vi "ReCalc.vi"(3 "Berechnen":bool, 4 "Datenspeicher":T3={"Fahrzeugdaten"="§$", "Auto-Pfad"="21.01.2021 18:54|N:\\Vespa-Prüfstand\\Läufe\\Test", "Rolle [Inkr/U]"=100, "Rollenumfang [m]"=0.942, "Rollenträgheit [kgm²]"=0.164, "Zündung [Imp/U]"=1.0, "Getriebe [1:]"=4.0, "Reifenumfang [m] "=1.222, "element"=3.988, "Gl. Mittelwert"=35, "Differenzenquotient"=12, "AFR, EGT"=1, "dT [s]"=0.02, "Strecke [m]"=150.92789069243696, "Lufttemperatur [°C]"=23.2, "Mv: n1 [1/min]"=1.0, "Luftdruck [mbar]"=100.34, "nRolle"=array[576 elements], "nWelle"=array[576 elements], "AFR"=[14.9, 14.9, 14.9, 14.9, 14.9, 14.9, 14.9, 14.9, 14.9, 14.9, 15.4, 15.4, 15.4, 15.4, 15.4, 14.8, 14.8, 14.8, 14.8, 14.8, 15.3, 15.3, 15.3, 15.3, 15.3, 15.2, 15.2, 15.2, 15.2, 15.2, 14.8, 14.8, 14.8, 14.8, 14.8, 15.0, 15.0, 15.0, 15.0, 15.0, 15.0, 15.0, 15.0, 15.0, 15.0, 15.0, 15.0, 15.0, 15.0, 15.0, 15.0, 15.0, 15.0, 15.0, 15.0, 15.4, 15.4, 15.4, 15.4, 15.4, 15.4, 15.4, 15.4, 15.4, 15.4, 14.9, 14.9, 14.9, 14.9, 14.9, 15.3, 15.3, 15.3, 15.3, 15.3, 15.0, 15.0, 15.0, 15.0, 15.0, 14.8, 14.8, 14.8, 14.8, 14.8, 15.2, 15.2, 15.2, 15.2, 15.2, 15.4, 15.4, 15.4, 15.4, 15.4, 15.1, 15.1, 15.1, 15.1, 15.1, 15.1, 15.1, 15.1, 15.1, 15.1, 15.1, 15.1, 15.1, 15.1, 15.1, 15.0, 15.0, 15.0, 15.0, 15.0, 15.0, 15.0, 15.0, 15.0, 15.0, 15.2, 15.2, 15.2, 15.2, 15.2, 15.1, 15.1, 15.1, 15.1, 15.1, 15.4, 15.4, 15.4, 15.4, 15.4, 15.1, 15.1, 15.1, 15.1, 15.1, 15.2, 15.2, 15.2, 15.2, 15.2, 14.8, 14.8, 14.8, 14.8, 14.8, 15.4, 15.4, 15.4, 15.4, 15.4, 15.0, 15.0, 15.0, 15.0, 15.0, 15.1, 15.1, 15.1, 15.1, 15.1, 15.0, 15.0, 15.0, 15.0, 15.0, 15.1, 15.1, 15.1, 15.1, 15.1, 14.9, 14.9, 14.9, 14.9, 14.9, 15.0, 15.0, 15.0, 15.0, 15.0, 15.2, 15.2, 15.2, 15.2, 15.2, 15.3, 15.3, 15.3, 15.3, 15.3, 15.1, 15.1, 15.1, 15.1, 15.1, 15.1, 15.1, 15.1, 15.1, 15.1, 14.9, 14.9, 14.9, 14.9, 14.9, 15.0, 15.0, 15.0, 15.0, 15.0, 15.3, 15.3, 15.3, 15.3, 15.3, 15.3, 15.3, 15.3, 15.3, 15.3, 15.1, 15.1, 15.1, 15.1, 15.1, 15.4, 15.4, 15.4, 15.4, 15.4, 15.0, 15.0, 15.0, 15.0, 15.0, 14.9, 14.9, 14.9, 14.9, 14.9, 15.0, 15.0, 15.0, 15.0, 15.0, 15.3, 15.3, 15.3, 15.3, 15.3, 15.0, 15.0, 15.0, 15.0, 15.0, 14.9, 14.9, 14.9, 14.9, 14.9, 14.9, 14.9, 14.9, 14.9, 14.9, 15.4, 15.4, 15.4, 15.4, 15.4, 15.1, 15.1, 15.1, 15.1, 15.1, 15.2, 15.2, 15.2, 15.2, 15.2, 15.2, 15.2, 15.2, 15.2, 15.2, 15.1, 15.1, 15.1, 15.1, 15.1, 15.4, 15.4, 15.4, 15.4, 15.4, 15.3, 15.3, 15.3, 15.3, 15.3, 14.9, 14.9, 14.9, 14.9, 14.9, 15.4, 15.4, 15.4, 15.4, 15.4, 15.1, 15.1, 15.1, 15.1, 15.1, 15.2, 15.2, 15.2, 15.2, 15.2, 15.2, 15.2, 15.2, 15.2, 15.2, 15.3, 15.3, 15.3, 15.3, 15.3, 14.9, 14.9, 14.9, 14.9, 14.9, 15.3, 15.3, 15.3, 15.3, 15.3, 14.9, 14.9, 14.9, 14.9, 14.9, 14.9, 14.9, 14.9, 14.9, 14.9, 15.1, 15.1, 15.1, 15.1, 15.1, 15.1, 15.1, 15.1, 15.1, 15.1, 15.3, 15.3, 15.3, 15.3, 15.3, 15.3, 15.3, 15.3, 15.3, 15.3, 15.0, 15.0, 15.0, 15.0, 15.0, 15.1, 15.1, 15.1, 15.1, 15.1, 15.2, 15.2, 15.2, 15.2, 15.2, 15.1, 15.1, 15.1, 15.1, 15.1, 15.4, 15.4, 15.4, 15.4, 15.4, 15.0, 15.0, 15.0, 15.0, 15.0, 15.4, 15.4, 15.4, 15.4, 15.4, 15.4, 15.4, 15.4, 15.4, 15.4, 15.1, 15.1, 15.1, 15.1, 15.1, 15.1, 15.1, 15.1, 15.1, 15.1, 15.0, 15.0, 15.0, 15.0, 15.0, 15.1, 15.1, 15.1, 15.1, 15.1, 15.1, 15.1, 15.1, 15.1, 15.1, 15.1, 15.1, 15.1, 15.1, 15.1, 15.2, 15.2, 15.2, 15.2, 15.2, 14.9, 14.9, 14.9, 14.9, 14.9, 15.2, 15.2, 15.2, 15.2, 15.2, 15.3, 15.3, 15.3, 15.3, 15.3, 15.3, 15.3, 15.3, 15.3, 15.3, 15.3, 15.3, 15.3, 15.3, 15.3, 14.9, 14.9, 14.9, 14.9, 14.9, 14.9, 14.9, 14.9, 14.9, 14.9, 15.1, 15.1, 15.1, 15.1, 15.1, 15.0, 15.0, 15.0, 15.0, 15.0, 15.4, 15.4, 15.4, 15.4, 15.4, 15.2, 15.2, 15.2, 15.2, 15.2, 15.1, 15.1, 15.1, 15.1, 15.1, 15.0, 15.0, 15.0, 15.0, 15.0, 15.1, 15.1, 15.1, 15.1, 15.1, 15.4, 15.4, 15.4, 15.4, 15.4, 15.0, 15.0, 15.0, 15.0, 15.0, 15.2, 15.2, 15.2, 15.2, 15.2, 14.9, 14.9, 14.9, 14.9, 14.9, 15.3, 15.3, 15.3, 15.3, 15.3, 14.9, 14.9, 14.9, 14.9, 14.9, 14.9, 14.9, 14.9, 14.9, 14.9, 15.0, 15.0, 15.0, 15.0, 15.0, 15.2, 15.2, 15.2, 15.2, 15.2, 15.0, 15.0, 15.0, 15.0, 15.0, 15.2, 15.2, 15.2, 15.2, 15.2, 15.2], "EGT"=array[576 elements], "Übersetzung ermitteln aus"=0, "[s]"=5.0, "Mv: M0 [Nm]"=0.0, "Mv: M1 [Nm]"=0.0, "n vom Gas [1/min]"=5000.0, "dT ungefiltert [s]"=array[576 elements], [], "Boolesch"=TRUE, "Serielle Schnittstelle"="", "nKuWe/nRolle 2"=3.988, "v vom Gas [km/h]"=40.0}) -> ()   [LabVIEW 2014]
uses:
  <vilib>/Utility/miscctls.llb/LVPointTypeDef.ctl
  <vilib>/Analysis/3filter.llb/IIR Filter (DBL).vi
  <vilib>/Analysis/NI_AALBase.lvlib
panel:
  in  "Resetskalierung Leistung":bool
  out "Y-Koord. Leistungsgraph-Reset-Button oben (567)":i32=567
  out "Y-Koord. Leistungsgraph-Reset-Button unten (782)":i32=782
  in  "Autoskalierung Leistung":bool
  in  "Resetskalierung AFR":bool
  in  "Autoskalierung AFR":bool
  out "EGT [°C]":dbl
  out "CursorAFR - Beschriftung":string="AFR"
  out "AFR":dbl format="%.1f"
  out "Fahrzeugdaten":string
  out "Ergebnis":string
  in  "Lambda":bool caption="Messung Klimadaten"
  in  "AFR, EGT":bool caption="Messung Klimadaten"
  out "Höhe Leistungs-Graph (646)":u32=646
  in  "title diagram":string
  out "Strecken":T1 {"Strecke7" scale=0.0..200.0; "Strecke6" scale=0.0..200.0; "Strecke5" scale=0.0..200.0; "Strecke4" scale=0.0..200.0; "Strecke3" scale=0.0..200.0; "Strecke2" scale=0.0..200.0; "Strecke1" max=600.0 scale=0.0..200.0}
  out "Dateiname":string
  out "Datum+Zeit":string="21.01.2021 18:54"
  out "Elementindex":dbl
  in  "Mv: M1 [Nm]":dbl min=0.0
  in  "Mv: M0 [Nm]":dbl min=0.0
  in  "Mv: n1 [1/min]":u16=1 min=1
  out "Überlagerung":bool
  out "CursorY2 - Beschriftung":string="M [Nm]"
  out "CursorX - Beschriftung":string="n [1/min]"
  out "M [Nm]":dbl format="%#.1f"
  out "P [PS]":dbl format="%#.1f"
  out "n [1/min]":dbl caption="n {1/min]" format="%#.0f"
  in  "v min [km/h]":dbl=40.0
  in  "Legende einblenden":bool=TRUE
  in  "Überlagern":bool
  out "Übersetzung ermitteln aus":T2(ring)
  in  "Speichern":bool
  out "circum. tire [m]":dbl=1.222
  out "gear ratio [1:]":dbl=4.0
  out "ignition [Imp/U]":dbl=1.0
  out "incre./rev.  [Inkr/U]":u16=100
  out "air pressure [mbar]":dbl=100.34
  out "air temp. [°C]":dbl=23.2
  in  "Stopp":bool
  in  "inertia dyno [kgm²]":dbl=0.164
  in  "mov. Average":u8=35
  in  "diff.quotient":u8=12
  in  "n min [1/min]":dbl=5000.0
  out "circum. dyno [m]":dbl=0.942 format="%.3f"
  out "gear ratio from:":dbl=3.988 format="%.2f"
  in  "Drucken":bool
  out "Pmax":string
  in  "Öffnen":bool
  out "korr":dbl=3.988
  out "XY-Graph":cluster{dbl[], dbl[]}[](graph)
  out "AFR,EGT-Graph":cluster{dbl[], dbl[]}[](graph)
  # "AFR / l &  EGT"
  # "Elementindex des Button \"Überlagern\" variierte zw. 24 und 25 nach Hinzufügen/Löschen anderer Objekte.\nKann hier abgefragt werden und im Case dann entsprechend eingetragen werden."
  # "AFR <> l"
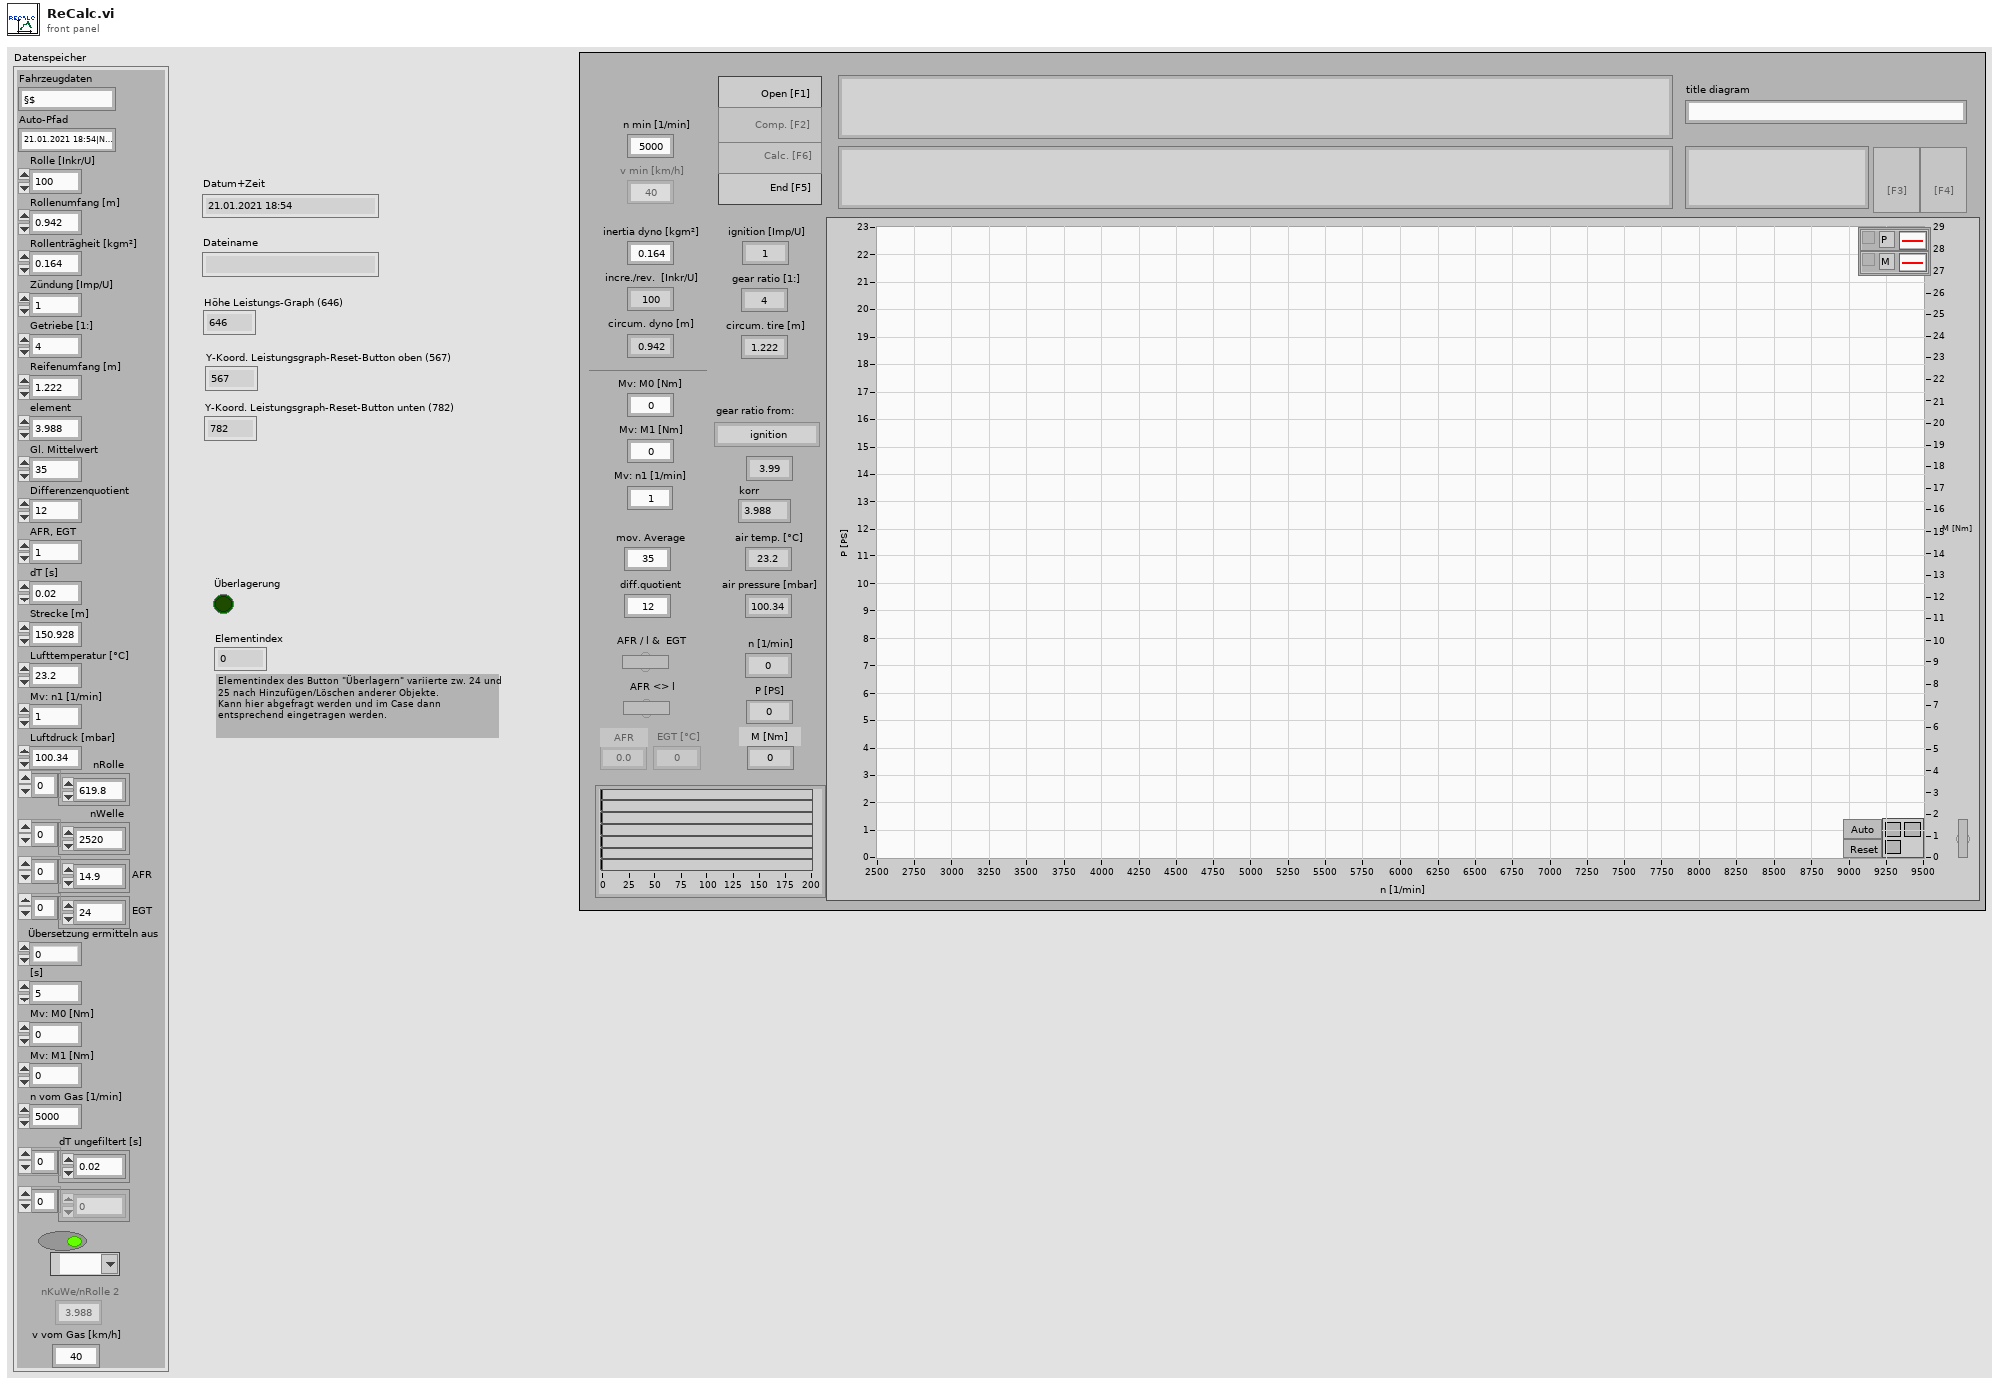
[diagram p1: front panel]
types:
  T1 = cluster{"Strecke1":dbl, "Strecke2":dbl, "Strecke3":dbl, "Strecke4":dbl, "Strecke5":dbl, "Strecke6":dbl, "Strecke7":dbl}
  T2 = enum8{"ignition ", "gear ratio & tire", "nCrank / nDyno", "vario [km/h]"}
  T3 = cluster{"Fahrzeugdaten":string, "Auto-Pfad":string, "Rolle [Inkr/U]":u16, "Rollenumfang [m]":dbl, "Rollenträgheit [kgm²]":dbl, "Zündung [Imp/U]":dbl, "Getriebe [1:]":dbl, "Reifenumfang [m] ":dbl, "element":dbl, "Gl. Mittelwert":u8, "Differenzenquotient":u8, "AFR, EGT":u8, "dT [s]":dbl, "Strecke [m]":dbl, "Lufttemperatur [°C]":dbl, "Mv: n1 [1/min]":dbl, "Luftdruck [mbar]":dbl, "nRolle":dbl[], "nWelle":dbl[], "AFR":dbl[], "EGT":dbl[], "Übersetzung ermitteln aus":u8, "[s]":dbl, "Mv: M0 [Nm]":dbl, "Mv: M1 [Nm]":dbl, "n vom Gas [1/min]":dbl, "dT ungefiltert [s]":dbl[], i32[], "Boolesch":bool, "Serielle Schnittstelle":refnum<visa-resource-name>, "nKuWe/nRolle 2":dbl, "v vom Gas [km/h]":dbl}
  T4 = typedef "LVPointTypeDef.ctl" = cluster{"Horizontal":i16, "Vertical":i16}
  T5 = enum8{"Enabled", "Disabled", "Disabled and Grayed Out"}
  T6 = cluster{"Fahrzeugdaten":string, "Auto-Pfad":string, "Rolle [Inkr/U]":u16, "Rollenumfang [m]":dbl, "Rollenträgheit [kgm²]":dbl, "Zündung [Imp/U]":dbl, "Getriebe [1:]":dbl, "Reifenumfang [m] ":dbl, "element":dbl, "Gl. Mittelwert":u8, "Differenzenquotient":u8, u8, "dT [s]":dbl, "Strecke [m]":dbl, "Lufttemperatur [°C]":dbl, "Mv: n1 [1/min]":dbl, "Luftdruck [mbar]":dbl, "nRolle":dbl[], "nWelle":dbl[], "AFR":dbl[], "EGT":dbl[], "Übersetzung ermitteln aus":u8, "[s]":dbl, "Mv: M0 [Nm]":dbl, "Mv: M1 [Nm]":dbl, "n vom Gas [1/min]":dbl, "dT-Array [s]":dbl[], i32[], "Boolesch":bool, "Serielle Schnittstelle":refnum<visa-resource-name>, "nKuWe/nRolle":dbl, "v vom Gas [km/h]":dbl}
  T7 = enum16{"Zündsignal", "Getriebe & Reifen", "nKuWe / nRolle", "Vario (km/h)"}
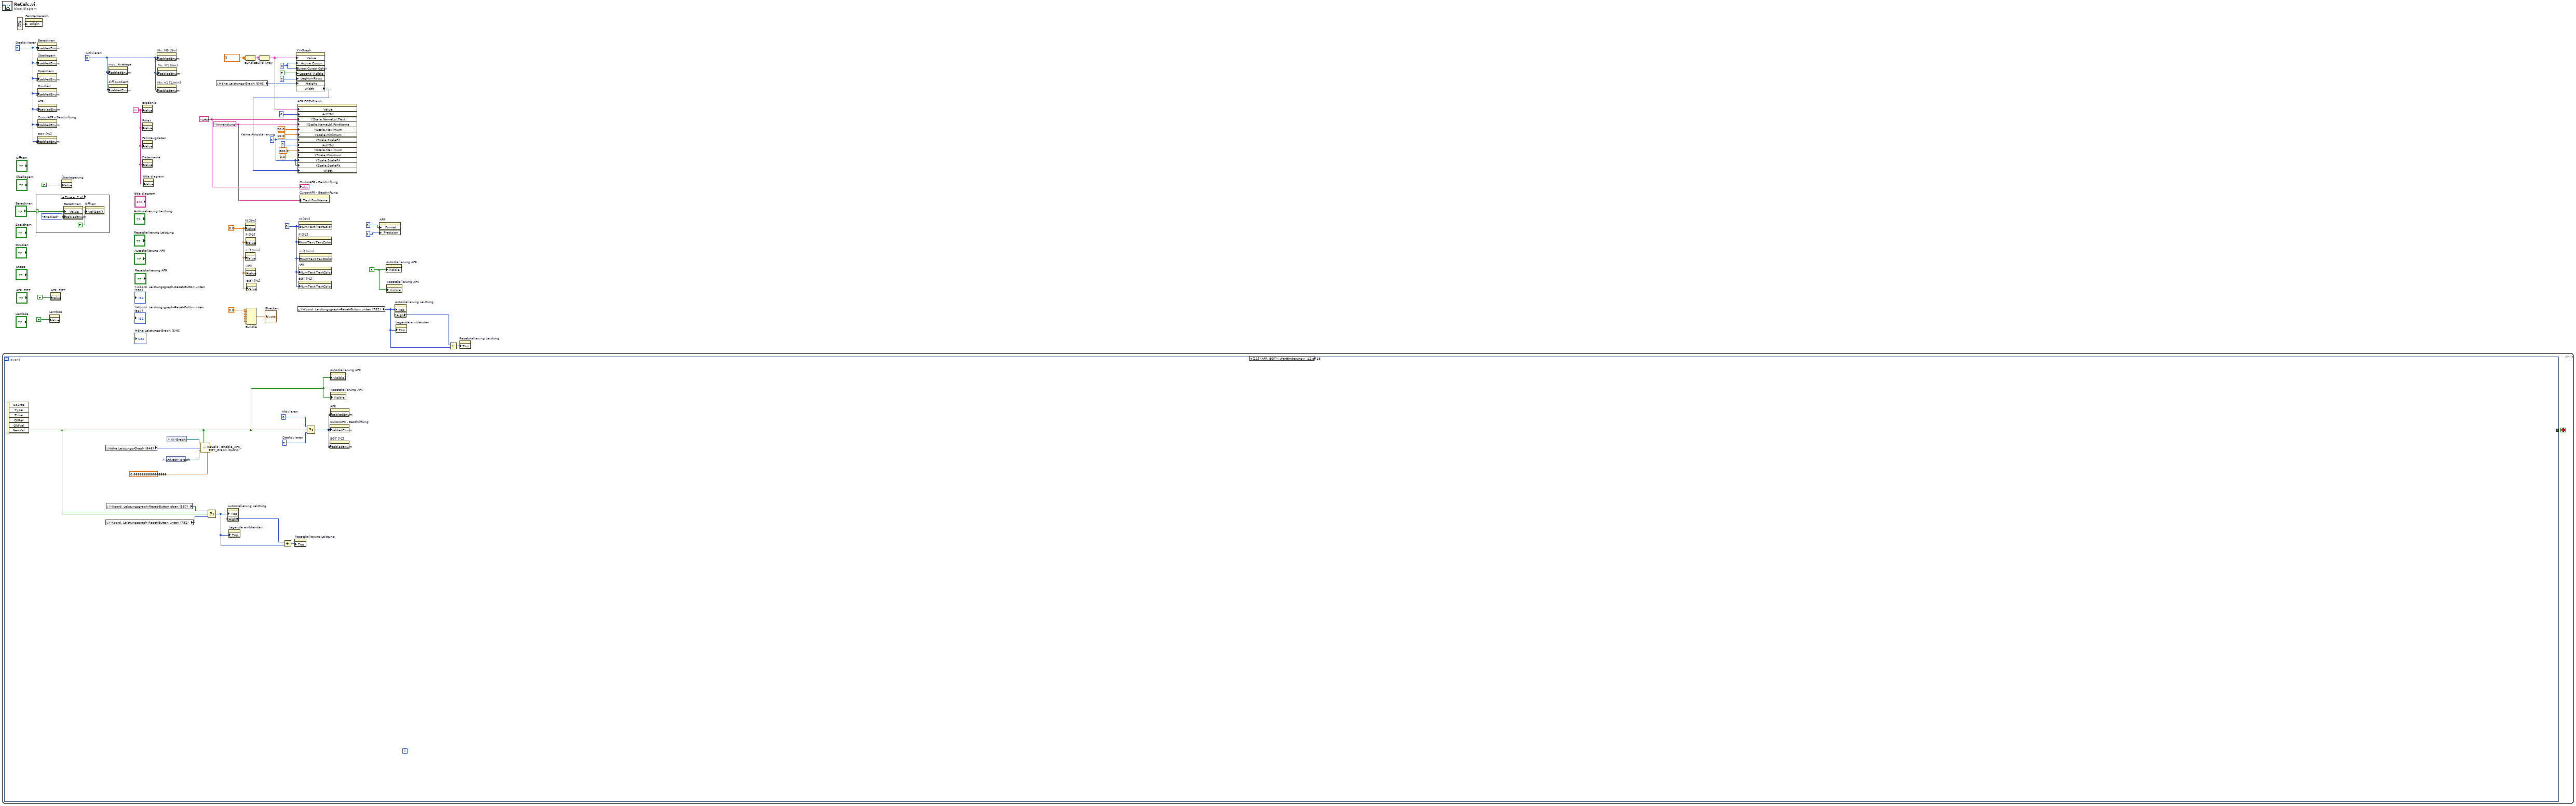
[diagram p0: block diagram]
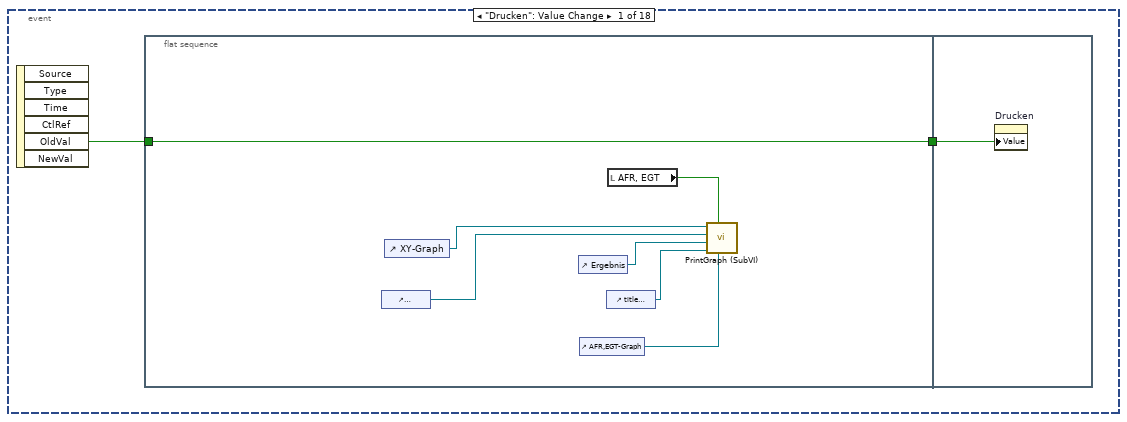
[diagram p3: hidden frame]
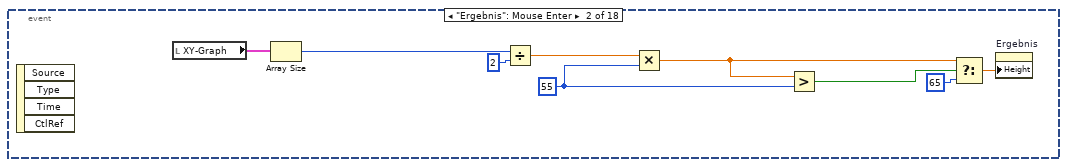
[diagram p4: hidden frame]
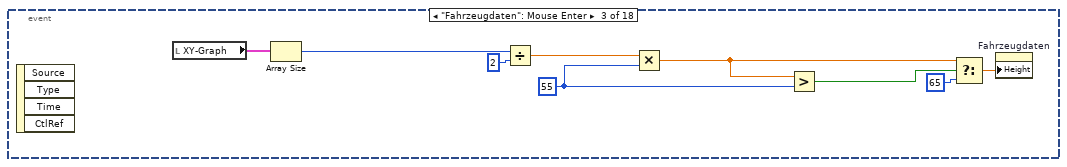
[diagram p5: hidden frame]
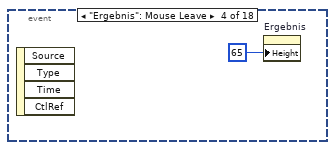
[diagram p6: hidden frame]
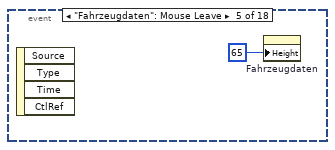
[diagram p7: hidden frame]
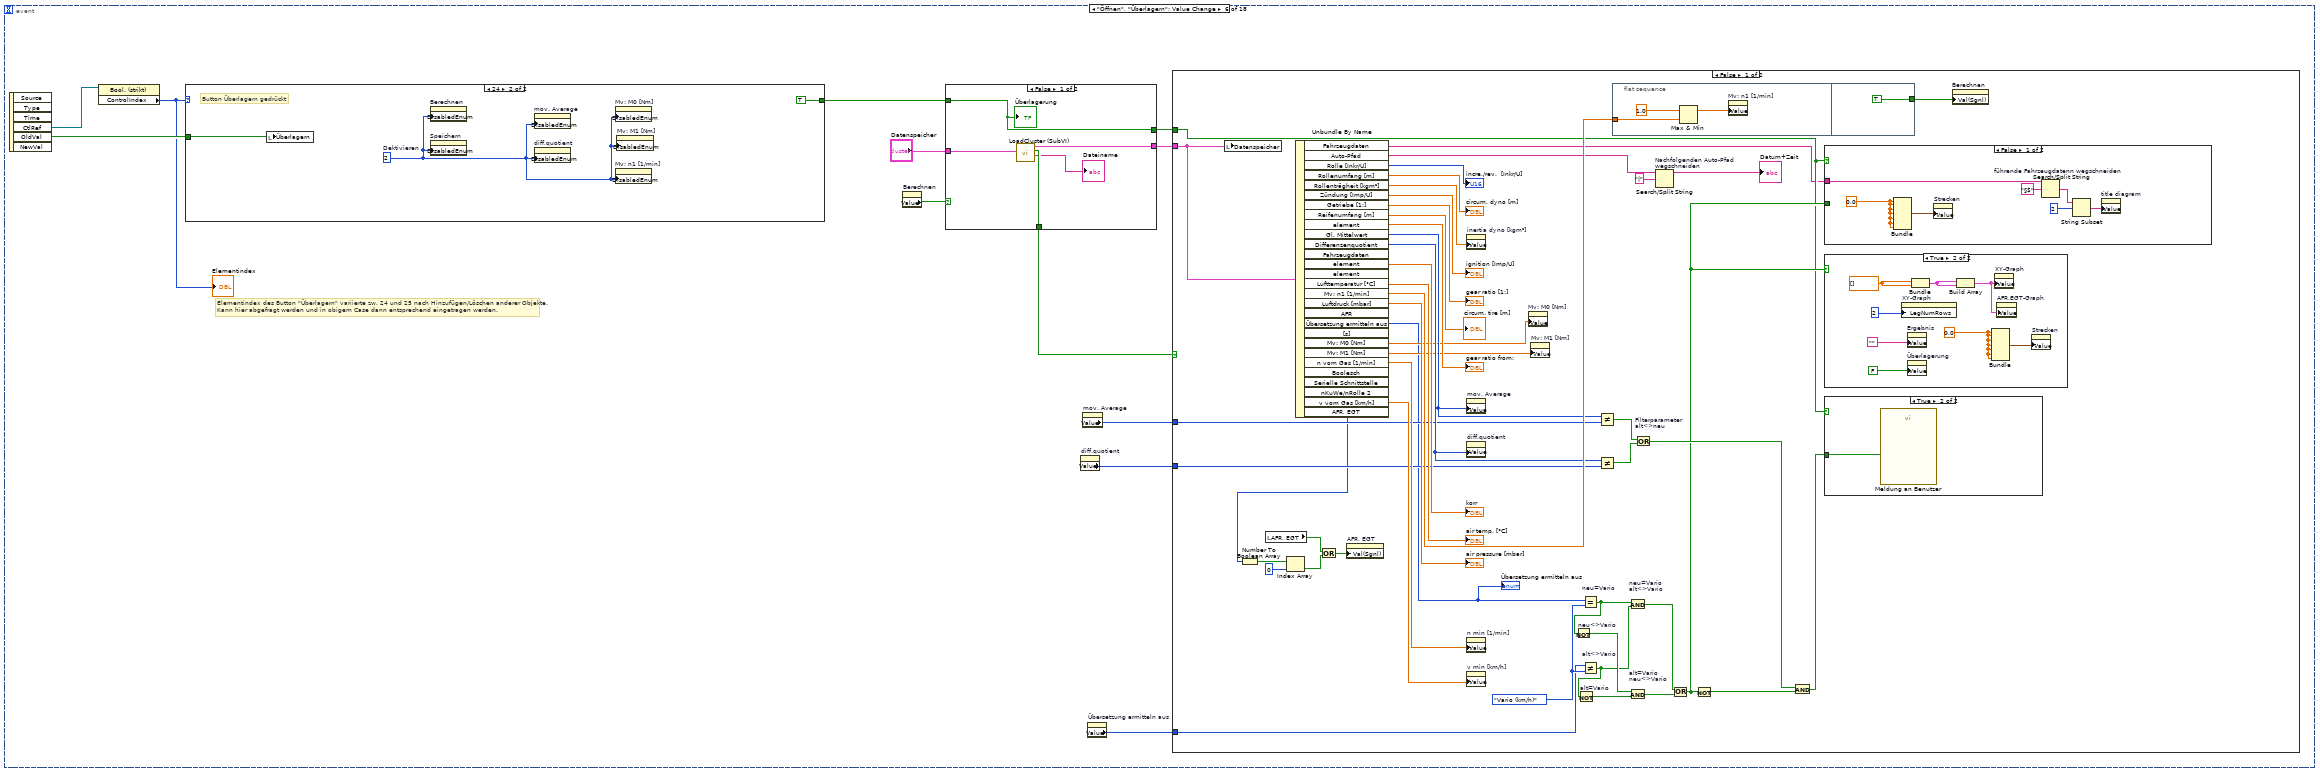
[diagram p8: hidden frame]
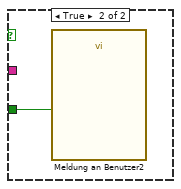
[diagram p10: hidden frame]
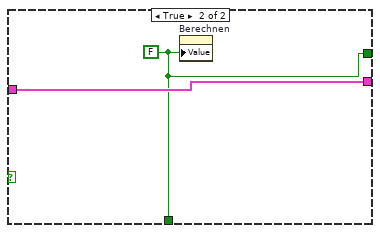
[diagram p13: hidden frame]
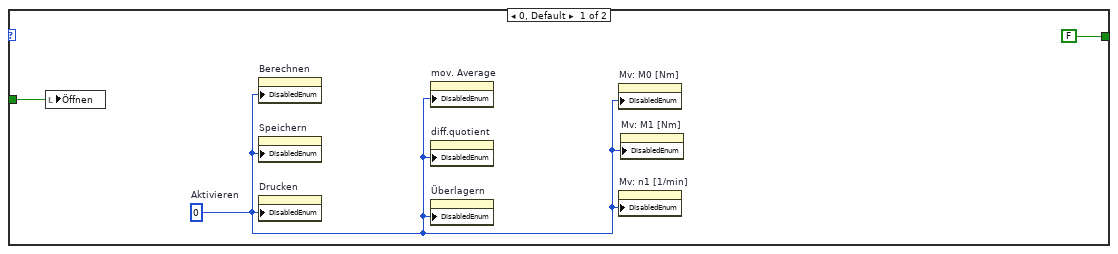
[diagram p14: hidden frame]
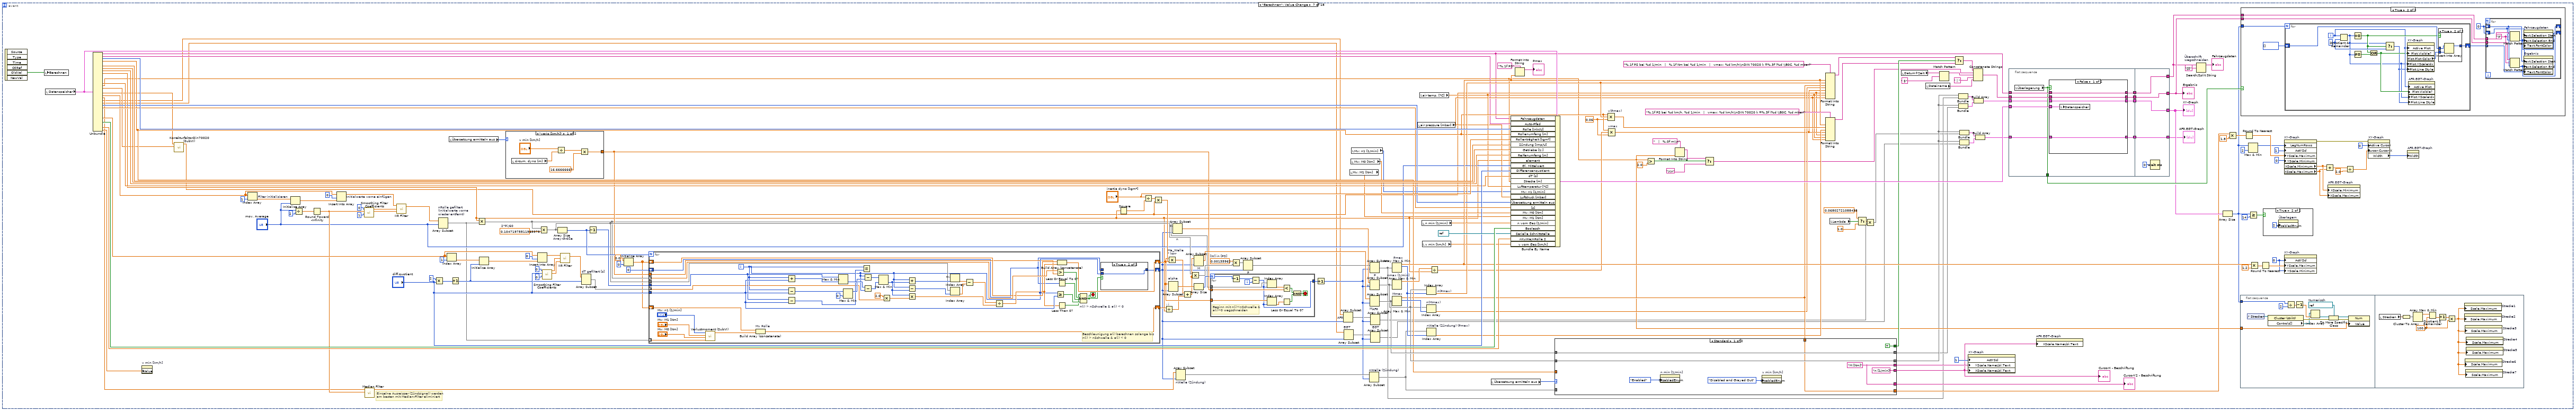
[diagram p15: hidden frame]
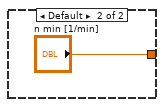
[diagram p16: hidden frame]
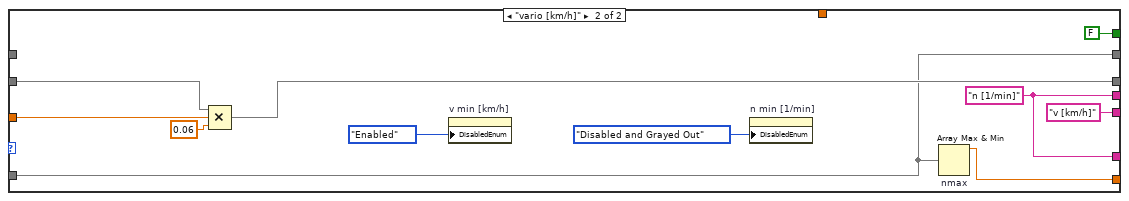
[diagram p17: hidden frame]
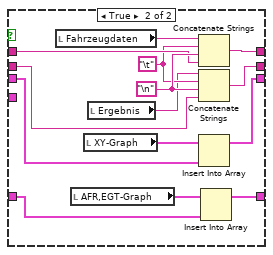
[diagram p19: hidden frame]
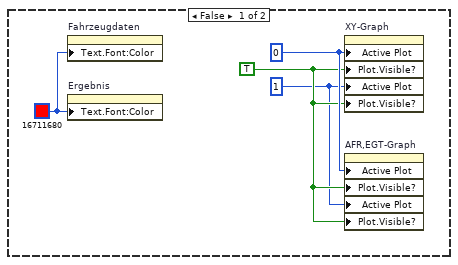
[diagram p20: hidden frame]
diagram:
  w5 = FALSE
  w11 = "Anwendung"
  w12 = "AFR"
  w14 = 0  # Keine Autoskalierung
  w27 = 0.0
  w31 = 0
  w8 = 0
  w10 = 0.0
  w33 = dbl[] []
  w29 = 0  # Aktivieren
  w9 = 2  # Deaktivieren
  w26 = ""
  n1 = while {
    stop <- w36 stop-if-true
    n2 = event shown="[11] \"AFR, EGT\": Wertänderung" {
      selector: _ -> [_ _ _ _ _ _ _ _ _ _ _ _ _ _ _ _ _ _]
      dyn-events: _ -> [_ _ _ _ _ _ _ _ _ _ _ _ _ _ _ _ _ _]
      timeout: _ -> [_ _ _ _ _ _ _ _ _ _ _ _ _ _ _ _ _ _]
      tunnel: [_ _ _ _ _ _ _ _ w518 _ _ _ _ _ _ _ _ _] -> w36
      event "Drucken": Value Change {
        n3 = event-data() -> ("OldVal"=w38:bool)  [unwired: 1 in, 5 out]
        n4 = flat-sequence {
          tunnel: [w45] -> w37
          tunnel: w38 -> [w45]
          tunnel: w37 -> [w46]
          frame #0 {
            n5 = control-ref of="Fahrzeugdaten"() -> (w43:refnum<vi>)
            n6 = control-ref of="XY-Graph"() -> (w44:refnum<vi>)
            n7 = control-ref of="Ergebnis"() -> (w42:refnum<vi>)
            n8 = control-ref of="AFR,EGT-Graph"() -> (w40:refnum<vi>)
            n9 = control-ref of="title diagram"() -> (w41:refnum<vi>)
            n10 = local read "AFR, EGT"() -> (w39:bool)
            n11 = call "PrintGraph (SubVI).vi"("AFR,EGT-Graph Ref"=w40, "AFR, EGT"=w39, "Überschrift"=w41, "Ergebnis"=w42, "Fahrzeugdaten"=w43, "P+M Graph Ref"=w44) -> ()  [unwired: 6 in]
          }
          frame #1 {
            n12 = property on="Drucken" class="Bool. (strikt)"("Value"=w46) -> ()  [unwired: 2 in, 2 out]
          }
        }
      }
      event "Ergebnis": Mouse Enter {
        w49 = u32 55 ("Größe:Höhe")
        n13 = event-data() -> ()  [unwired: 1 in, 4 out]
        n14 = local read "XY-Graph"() -> (w55:cluster{dbl[], dbl[]}[])
        n15 = Array Size(array=w55) -> (size(s)=w54:i32)
        n16 = Divide(x=w54, y=2) -> (x/y=w52:dbl)
        n17 = Multiply(x=w52, y=w49) -> (x*y=w50:dbl)
        n18 = Greater?(x=w50, y=w49) -> (0:w51:bool)
        n19 = Select(t=w50, s=w51, f=u32 65 ("Größe:Höhe")) -> (s? t:f=w48:dbl)
        n20 = property on="Ergebnis" class="Str"("Height"=w48) -> ()  [unwired: 2 in, 2 out]
      }
      event "Fahrzeugdaten": Mouse Enter {
        w58 = u32 55 ("Größe:Höhe")
        n21 = event-data() -> ()  [unwired: 1 in, 4 out]
        n22 = local read "XY-Graph"() -> (w64:cluster{dbl[], dbl[]}[])
        n23 = Array Size(array=w64) -> (size(s)=w63:i32)
        n24 = Divide(x=w63, y=2) -> (x/y=w61:dbl)
        n25 = Multiply(x=w61, y=w58) -> (x*y=w59:dbl)
        n26 = Greater?(x=w59, y=w58) -> (0:w60:bool)
        n27 = Select(t=w59, s=w60, f=u32 65 ("Größe:Höhe")) -> (s? t:f=w57:dbl)
        n28 = property on="Fahrzeugdaten" class="Str"("Height"=w57) -> ()  [unwired: 2 in, 2 out]
      }
      event "Ergebnis": Mouse Leave {
        n29 = event-data() -> ()  [unwired: 1 in, 4 out]
        n30 = property on="Ergebnis" class="Str"("Height"=u32 65 ("Größe:Höhe")) -> ()  [unwired: 2 in, 2 out]
      }
      event "Fahrzeugdaten": Mouse Leave {
        n31 = event-data() -> ()  [unwired: 1 in, 4 out]
        n32 = property on="Fahrzeugdaten" class="Str"("Height"=u32 65 ("Größe:Höhe")) -> ()  [unwired: 2 in, 2 out]
      }
      event "Öffnen", "Überlagern": Value Change {
        # "Elementindex des Button \"Überlagern\" variierte zw. 24 und 25 nach Hinzufügen/Löschen anderer Objekte.\nKann hier abgefragt werden und in obigem Case dann entsprechend eingetragen werden."
        n33 = event-data() -> ("CtlRef"=w77:refnum<vi>, "OldVal"=w68:bool)  [unwired: 1 in, 4 out]
        n34 = property class="Bool. (strikt)"(reference=w77) -> ("ControlIndex"=w67:i32)  [unwired: 1 in, 2 out]
        "Elementindex" <- w67
        n35 = case shown="24" w67 {
          tunnel: w68 -> [w156 w159]
          tunnel: [FALSE ("Überlagerung") TRUE ("Überlagerung")] -> w76
          frame 0, Default {
            w154 = 0  # Aktivieren
            n36 = local write "Öffnen"(w156) -> ()
            n37 = property on="Berechnen" class="Bool. (strikt)"("DisabledEnum"=w154) -> ()  [unwired: 2 in, 2 out]
            n38 = property on="Speichern" class="Bool. (strikt)"("DisabledEnum"=w154) -> ()  [unwired: 2 in, 2 out]
            n39 = property on="Drucken" class="Bool. (strikt)"("DisabledEnum"=w154) -> ()  [unwired: 2 in, 2 out]
            n40 = property on="mov. Average" class="DigWert (strikt)"("DisabledEnum"=w154) -> ()  [unwired: 2 in, 2 out]
            n41 = property on="diff.quotient" class="DigWert (strikt)"("DisabledEnum"=w154) -> ()  [unwired: 2 in, 2 out]
            n42 = property on="Überlagern" class="Bool. (strikt)"("DisabledEnum"=w154) -> ()  [unwired: 2 in, 2 out]
            n43 = property on="Mv: M0 [Nm]" class="DigWert (strikt)"("DisabledEnum"=w154) -> ()  [unwired: 2 in, 2 out]
            n44 = property on="Mv: n1 [1/min]" class="DigWert (strikt)"("DisabledEnum"=w154) -> ()  [unwired: 2 in, 2 out]
            n45 = property on="Mv: M1 [Nm]" class="DigWert (strikt)"("DisabledEnum"=w154) -> ()  [unwired: 2 in, 2 out]
          }
          frame 24 {
            w157 = 2  # Dektivieren
            # "Button Überlagern gedrückt"
            n46 = local write "Überlagern"(w159) -> ()
            n47 = property on="Berechnen" class="Bool. (strikt)"("DisabledEnum"=w157) -> ()  [unwired: 2 in, 2 out]
            n48 = property on="Speichern" class="Bool. (strikt)"("DisabledEnum"=w157) -> ()  [unwired: 2 in, 2 out]
            n49 = property on="mov. Average" class="DigWert (strikt)"("DisabledEnum"=w157) -> ()  [unwired: 2 in, 2 out]
            n50 = property on="diff.quotient" class="DigWert (strikt)"("DisabledEnum"=w157) -> ()  [unwired: 2 in, 2 out]
            n51 = property on="Mv: M0 [Nm]" class="DigWert (strikt)"("DisabledEnum"=w157) -> ()  [unwired: 2 in, 2 out]
            n52 = property on="Mv: n1 [1/min]" class="DigWert (strikt)"("DisabledEnum"=w157) -> ()  [unwired: 2 in, 2 out]
            n53 = property on="Mv: M1 [Nm]" class="DigWert (strikt)"("DisabledEnum"=w157) -> ()  [unwired: 2 in, 2 out]
          }
        }
        n54 = property on="Berechnen" class="Bool. (strikt)"() -> ("Value"=w75:bool)  [unwired: 2 in, 2 out]
        n55 = case shown="False" w75 {
          tunnel: "Datenspeicher" -> [w150 w153]
          tunnel: w76 -> [w151 _]
          tunnel: [w149 w153] -> w73
          tunnel: [w151 w152] -> w74
          tunnel: [w148 w152] -> w72
          frame False {
            n56 = call "LoadCluster (SubVI).vi"("Datenspeicher"=w150) -> ("Dateiname"=→"Dateiname":string, "cancelled"=w148:bool, "Value"=w149:T6)  [unwired: 8 in]
            "Überlagerung" <- w151
          }
          frame True {
            w152 = FALSE
            n57 = property on="Berechnen" class="Bool. (strikt)"("Value"=w152) -> ()  [unwired: 2 in, 2 out]
          }
        }
        n58 = property on="diff.quotient" class="DigWert (strikt)"() -> ("Value"=w70:u8)  [unwired: 2 in, 2 out]
        n59 = property on="mov. Average" class="DigWert (strikt)"() -> ("Value"=w69:u8)  [unwired: 2 in, 2 out]
        n60 = property on="Übersetzung ermitteln aus" class="Enum (strikt)"() -> ("Value"=w71:T2)  [unwired: 2 in, 2 out]
        n61 = case shown="False" w72 {
          tunnel: w74 -> [w103 _]
          tunnel: w73 -> [w105 _]
          tunnel: w71 -> [w96 _]
          tunnel: w70 -> [w95 _]
          tunnel: w69 -> [w94 _]
          frame False {
            w97 = T7."Vario (km/h)"
            n62 = local write "Datenspeicher"(w105) -> ()
            n63 = local read "AFR, EGT"() -> (w82:bool)
            n64 = Unbundle By Name(w105) -> ("Fahrzeugdaten"=w86:string, "Auto-Pfad"=w89:string, "Rolle [Inkr/U]"=→"incre./rev.  [Inkr/U]":u16, "Rollenumfang [m]"=→"circum. dyno [m]":dbl, "Rollenträgheit [kgm²]"=w117:dbl, "Zündung [Imp/U]"=→"ignition [Imp/U]":dbl, "Getriebe [1:]"=→"gear ratio [1:]":dbl, "Reifenumfang [m]"=→"circum. tire [m]":dbl, "element"=→"gear ratio from:":dbl, "Gl. Mittelwert"=w114:u8, "Differenzenquotient"=w113:u8, "element"=→"korr":dbl, "Lufttemperatur [°C]"=→"air temp. [°C]":dbl, "Mv: n1 [1/min]"=w124:dbl, "Luftdruck [mbar]"=→"air pressure [mbar]":dbl, "Übersetzung ermitteln aus"=w79:u8, "Mv: M0 [Nm]"=w91:dbl, "Mv: M1 [Nm]"=w90:dbl, "n vom Gas [1/min]"=w125:dbl, "v vom Gas [km/h]"=w109:dbl, "AFR, EGT"=w83:u8)  [unwired: 7 out]
            "Übersetzung ermitteln aus" <- w79
            n65 = Number To Boolean Array(number=w83) -> (Boolean array=w85:bool[])
            n66 = Index Array(array=w85, index=0) -> (element=w81:bool)
            n67 = Or(x=w82, y=w81) -> (x .or. y?=w80:bool)
            n68 = property on="AFR, EGT" class="Bool. (strikt)"("Val(Sgnl)"=w80) -> ()  [unwired: 2 in, 2 out]
            n69 = property on="inertia dyno [kgm²]" class="DigWert (strikt)"("Value"=w117) -> ()  [unwired: 2 in, 2 out]
            n70 = property on="mov. Average" class="DigWert (strikt)"("Value"=w114) -> ()  [unwired: 2 in, 2 out]
            n71 = property on="diff.quotient" class="DigWert (strikt)"("Value"=w113) -> ()  [unwired: 2 in, 2 out]
            n72 = property on="n min [1/min]" class="DigWert (strikt)"("Value"=w125) -> ()  [unwired: 2 in, 2 out]
            n73 = property on="v min [km/h]" class="DigWert (strikt)"("Value"=w109) -> ()  [unwired: 2 in, 2 out]
            n74 = property on="Mv: M0 [Nm]" class="DigWert (strikt)"("Value"=w91) -> ()  [unwired: 2 in, 2 out]
            n75 = property on="Mv: M1 [Nm]" class="DigWert (strikt)"("Value"=w90) -> ()  [unwired: 2 in, 2 out]
            n76 = Equal? "neu=Vario"(x=w79, y=w97) -> (x = y?=w98:bool)
            n77 = Not "neu<>Vario"(x=w98) -> (.not. x?=w99:bool)
            n78 = Not Equal? "alt<>Vario"(x=w96, y=w97) -> (x != y?=w92:bool)
            n79 = Not "alt=Vario"(x=w92) -> (.not. x?=w93:bool)
            n80 = Not Equal?(x=w114, y=w94) -> (x != y?=w112:bool)
            n81 = Not Equal?(x=w113, y=w95) -> (x != y?=w111:bool)
            n82 = flat-sequence {
              tunnel: w124 -> [w145]
              tunnel: [TRUE] -> w106
              frame #0 {
                n83 = Max & Min(x=1.0, y=w145) -> (max(x,y)=w143:dbl)  [unwired: 1 out]
                n84 = property on="Mv: n1 [1/min]" class="DigWert (strikt)"("Value"=w143) -> ()  [unwired: 2 in, 2 out]
              }
              frame #1 {
              }
            }
            n85 = And "neu=Vario\nalt<>Vario"(x=w98, y=w92) -> (x .and. y?=w101:bool)
            n86 = And "alt=Vario\nneu<>Vario"(x=w99, y=w93) -> (x .and. y?=w100:bool)
            n87 = Or "Filterparameter\nalt<>neu"(x=w112, y=w111) -> (x .or. y?=w107:bool)
            n88 = Search/Split String "Nachfolgenden Auto-Pfad wegschneiden"(string=w89, search string/char (-)="|") -> (substring before match=→"Datum+Zeit":string)  [unwired: 1 in, 2 out]
            n89 = Or(x=w101, y=w100) -> (x .or. y?=w104:bool)
            n90 = Not(x=w104) -> (.not. x?=w108:bool)
            n91 = And(x=w107, y=w108) -> (x .and. y?=w102:bool)
            n92 = case shown="True" w104 {
              frame False {
              }
              frame True {
                w128 = 0.0
                w129 = dbl[] []
                n93 = property on="XY-Graph" class="XYGraph (strikt)"("LegNumRows"=2) -> ()  [unwired: 2 in, 2 out]
                n94 = property on="Ergebnis" class="Str"("Value"="") -> ()  [unwired: 2 in, 2 out]
                n95 = property on="Überlagerung" class="Bool. (strikt)"("Value"=FALSE) -> ()  [unwired: 2 in, 2 out]
                n96 = Bundle(w129, w129) -> (w130:cluster{dbl[], dbl[]})  [unwired: 1 in]
                n97 = Build Array(w130, w130) -> (w126:cluster{dbl[], dbl[]}[])
                n98 = Bundle(w128, w128, w128, w128, w128, w128, w128) -> (w127:cluster{dbl, dbl, dbl, dbl, dbl, dbl, dbl})  [unwired: 1 in]
                n99 = property on="XY-Graph" class="XYGraph (strikt)"("Value"=w126) -> ()  [unwired: 2 in, 2 out]
                n100 = property on="AFR,EGT-Graph" class="XYGraph (strikt)"("Value"=w126) -> ()  [unwired: 2 in, 2 out]
                n101 = property on="Strecken" class="Cluster (strikt)"("Value"=w127) -> ()  [unwired: 2 in, 2 out]
              }
            }
            n102 = case shown="True" w103 {
              tunnel: w102 -> [_ w142]
              frame False {
              }
              frame True {
                n103 = call "Meldung an Benutzer"("Enable"=w142) -> ()  [unwired: 9 in, 2 out]
              }
            }
            n104 = case shown="False" w103 {
              tunnel: w104 -> [_ w141]
              tunnel: w86 -> [w134 _]
              frame False {
                w139 = 0.0
                n105 = Bundle(w139, w139, w139, w139, w139, w139, w139) -> (w140:cluster{dbl, dbl, dbl, dbl, dbl, dbl, dbl})  [unwired: 1 in]
                n106 = property on="Strecken" class="Cluster (strikt)"("Value"=w140) -> ()  [unwired: 2 in, 2 out]
                n107 = Search/Split String "führende Fahrzeugdatenn wegschneiden"(string=w134, search string/char (-)="§$") -> (match + rest of string=w137:string)  [unwired: 1 in, 2 out]
                n108 = String Subset(string=w137, offset (0)=2) -> (substring=w138:string)  [unwired: 1 in]
                n109 = property on="title diagram" class="Str"("Value"=w138) -> ()  [unwired: 2 in, 2 out]
              }
              frame True {
                n110 = call "Meldung an Benutzer2"("Enable"=w141) -> ()  [unwired: 9 in, 2 out]
              }
            }
            n111 = property on="Berechnen" class="Bool. (strikt)"("Val(Sgnl)"=w106) -> ()  [unwired: 2 in, 2 out]
          }
          frame True {
          }
        }
      }
      event "Berechnen": Value Change {
        w227 = 0.06
        w262 = 0
        w338 = 0.00135962  # [W] in [PS]
        w344 = 0.10471975511965978  # 2*Pi/60
        # "Einzelne Ausreisser (Zündsignal) werden\nam besten mit Median-Filter eliminiert"
        n112 = event-data() -> ("OldVal"=w311:bool)  [unwired: 1 in, 5 out]
        n113 = local write "Berechnen"(w311) -> ()
        n114 = local read "Datenspeicher"() -> (w320:T3)
        n115 = Unbundle(w320) -> ("Fahrzeugdaten"=w189:string, "Auto-Pfad"=w218:string, "Rolle [Inkr/U]"=w319:u16, "Rollenumfang [m]"=w229:dbl, "Zündung [Imp/U]"=w316:dbl, "Getriebe [1:]"=w315:dbl, "Reifenumfang [m]"=w314:dbl, "element"=w211:dbl, "dT [s]"=w286:dbl, "Strecke [m]"=w190:dbl, "Lufttemperatur [°C]"=w203:dbl, "Luftdruck [mbar]"=w202:dbl, "nRolle"=w164:dbl[], "nWelle"=w235:dbl[], "AFR"=w162:dbl[], "EGT"=w163:dbl[], "Übersetzung ermitteln aus"=w246:u8, "[s]"=w312:dbl, "dT ungefiltert [s]"=w245:dbl[], "Boolesch"=w317:bool, "nKuWe/nRolle 2"=w270:dbl, "v vom Gas [km/h]"=w267:dbl)  [unwired: 10 out]
        n116 = property on="v min [km/h]" class="DigWert (strikt)"("Value"=w267) -> ()  [unwired: 2 in, 2 out]
        n117 = call "KorrekturfaktorDin70020 (SubVI).vi"("Lufttemperatur [°C]"=w203, "Luftdruck [mbar]"=w202) -> ("Korrekturfaktor"=w201:dbl)  [unwired: 9 in]
        n118 = Index Array "Filter initialisieren"(array=w164, index=1) -> (element=w324:dbl)
        n119 = Initialize Array(w324, "mov. Average") -> (w325:dbl[])
        n120 = Divide(x="mov. Average", y=2) -> (x/y=w346:dbl)
        n121 = Round Toward -Infinity(1:w346) -> (0:w237:dbl)
        n122 = Insert Into Array "Initialwerte vorne einfügen"(array=w164, index=0, new element=w325) -> (w244:dbl[])
        n123 = call <vilib>:"Smoothing Filter Coefficients.vi"("shape"=1, "half-width"=w237, "type"=0) -> ("forward coefficients"=w247:dbl[], "reverse coefficients"=w248:dbl[])  [unwired: 6 in, 1 out]
        n124 = call <vilib>:"Median Filter.vi"("left rank"=w237, "X"=w235) -> ("Filtered X"=w234:dbl[])  [unwired: 8 in, 1 out]
        n125 = call-poly <vilib>:"IIR Filter.vi"("Forward Coefficients"=w247, "Reverse Coefficients"=w248, "X"=w244) -> ("Filtered X"=w322:dbl[])  [unwired: 1 in, 1 out]
        n126 = Multiply(x=2, y="diff.quotient") -> (x*y=w294:i32)
        n127 = Array Subset "nRolle gefiltert\n(Initialwerte vorne \nwieder entfernt)"(array=w322, index="mov. Average") -> (w214:dbl[])  [unwired: 1 in]
        n128 = Index Array(array=w245, index=1 ("Index")) -> (element=w292:dbl)
        n129 = local read "Übersetzung ermitteln aus"() -> (w265:T2)
        n130 = Increment(x=w294) -> (x+1=w287:i32)
        n131 = Multiply(x=w211, y=w214) -> (x*y=w239:dbl[])
        n132 = Initialize Array(w292, w287) -> (w290:dbl[])
        n133 = case shown="\"vario [km/h]\"" w265 {
          tunnel: [w371 "n min [1/min]"] -> w266
          frame "vario [km/h]" {
            n134 = local read "circum. dyno [m]"() -> (w372:dbl)
            n135 = Divide(x="v min [km/h]", y=w372) -> (x/y=w370:dbl)
            n136 = Multiply(x=w370, y=16.66666667) -> (x*y=w371:dbl)
          }
          frame Default {
          }
        }
        n137 = Insert Into Array(array=w245, index=0 ("Index"), new element=w290) -> (w289:dbl[])
        n138 = Multiply(x=w239, y=w344) -> (x*y=w282:dbl[])
        n139 = call <vilib>:"Smoothing Filter Coefficients.vi"("shape"=0, "half-width"="diff.quotient", "type"=0) -> ("forward coefficients"=w297:dbl[], "reverse coefficients"=w298:dbl[])  [unwired: 6 in, 1 out]
        n140 = Array Size "Array-Größe"(array=w282) -> (size(s)=w342:i32)
        n141 = call-poly <vilib>:"IIR Filter.vi"("Forward Coefficients"=w297, "Reverse Coefficients"=w298, "X"=w289) -> ("Filtered X"=w288:dbl[])  [unwired: 1 in, 1 out]
        n142 = Array Subset "dT gefiltert [s]"(array=w288, index=w287) -> (w243:dbl[])  [unwired: 1 in]
        n143 = Decrement(x=w342) -> (x-1=w343:i32)
        n144 = Initialize Array(0.0 ("y"), 0) -> (w213:dbl[])
        n145 = for {
          N: w342 -> [_]
          tunnel: "diff.quotient" -> [w494]
          tunnel: w282 -> [w483]
          tunnel: w343 -> [w493]
          shift-right: [w498] -> w283
          shift-left: w213 -> [w482]
          tunnel: w239 -> [w496] mode=indexing
          tunnel: w266 -> [w480]
          shift-right: [w487] -> w176
          shift-left: 0 -> [w479]
          tunnel: w243 -> [w484] mode=indexing
          tunnel: w214 -> [w478] mode=indexing
          shift-right: [w472] -> w212
          shift-left: w213 -> [w473]
          i -> [w481]
          stop <- w488 stop-if-true
          # "Beschleunigung a(i) berechnen solange bis\nn(i) > nSchwelle & a(i) < 0"
          n146 = call "Verlustmoment (SubVI).vi"("n [1/min"=w478, "Verlustmoment M0 [Nm] bei n = 0"="Mv: M0 [Nm]", "Verlustmoment M1 [Nm] bei n1"="Mv: M1 [Nm]", "Rollendrehzahl n1 [1/min]"="Mv: n1 [1/min]") -> ("Mv"=w474:dbl)  [unwired: 7 in]
          n147 = Build Array (concatenate) "Mv Rolle"(w473, w474) -> (w472:dbl[])
          n148 = Add(x=w481, y=w494) -> (x+y=w506:i32)
          n149 = Subtract(x=w481, y=w494) -> (x-y=w512:i32)
          n150 = Subtract(x=w493, y=w494) -> (x-y=w495:i32)
          n151 = Max & Min(x=w493, y=w506) -> (min(x,y)=w507:i32)  [unwired: 1 out]
          n152 = Max & Min(x=w512, y=0) -> (max(x,y)=w510:i32)  [unwired: 1 out]
          n153 = Less Or Equal?(x=w481, y=w495) -> ()  [unwired: 1 out]
          n154 = Subtract(x=w481, y=w510) -> (x-y=w509:i32)
          n155 = Subtract(x=w507, y=w481) -> (x-y=w508:i32)
          n156 = Max & Min(x=w509, y=w508) -> (min(x,y)=w500:i32)  [unwired: 1 out]
          n157 = Multiply(x=2.0, y=w484) -> (x*y=w485:dbl)
          n158 = Add(x=w481, y=w500) -> (x+y=w505:i32)
          n159 = Subtract(x=w481, y=w500) -> (x-y=w504:i32)
          n160 = Multiply(x=w500, y=w485) -> (x*y=w499:dbl)
          n161 = Index Array(array=w483, index=w505) -> (element=w502:dbl)
          n162 = Index Array(array=w483, index=w504) -> (element=w503:dbl)
          n163 = Subtract(x=w502, y=w503) -> (x-y=w501:dbl)
          n164 = Divide(x=w501, y=w499) -> (x/y=w492:dbl)
          n165 = Greater?(x=w496, y=w480) -> (0:w497:bool)
          n166 = Greater Or Equal?(x=w481, y=w494) -> (x >= y?=w491:bool)
          n167 = Build Array (concatenate)(w482, w492) -> (w498:dbl[])
          n168 = Less Or Equal To 0?(x=w479) -> (x <= 0?=w489:bool)
          n169 = Less Than 0?(x=w492) -> (x < 0?=w490:bool)
          n170 = Compound Arithmetic op=AND "n(i) > nSchwelle & a(i) < 0"(w490, w497, w489, w491) -> (w488:bool)
          n171 = case shown="True" w488 {
            tunnel: w481 -> [_ w514]
            tunnel: [w513 w514] -> w487
            tunnel: w479 -> [w513 _]
            frame False {
            }
            frame True {
            }
          }
        }
        n172 = Square(x=w211) -> (x^2=w339:dbl)
        n173 = Divide(x="inertia dyno [kgm²]", y=w339) -> (x/y=w336:dbl)
        n174 = Multiply(x=w336, y=w201) -> (x*y=w335:dbl)
        n175 = Divide ": i"(x=w212, y=w211) -> (x/y=w210:dbl[])
        n176 = Multiply "Ma_Welle\n* korr"(x=w283, y=w335) -> (x*y=w208:dbl[])
        n177 = Array Subset "alpha"(array=w283, length=w176) -> (w333:dbl[])  [unwired: 1 in]
        n178 = Array Subset "n"(array=w239, length=w176) -> (w242:dbl[])  [unwired: 1 in]
        n179 = Array Subset "nWelle (Zündung)"(array=w234, length=w176) -> (w238:dbl[])  [unwired: 1 in]
        n180 = Add(x=w208, y=w210) -> (x+y=w209:dbl[])
        n181 = Multiply(x=w282, y=w209) -> (x*y=w337:dbl[])
        n182 = Array Subset "M"(array=w209, length=w176) -> (w285:dbl[])  [unwired: 1 in]
        n183 = Array Size(array=w333) -> (size(s)=w240:i32)
        n184 = for {
          N: w240 -> [w471]
          tunnel: w283 -> [w468]
          tunnel: w239 -> [w467]
          tunnel: w266 -> [w466]
          tunnel: [w464] -> w331
          i -> [w460]
          stop <- w465 stop-if-true
          # "Beginn mit n(i)<nSchwelle &  a(i)<0 wegschneiden"
          n185 = Decrement(x=w471) -> (x-1=w470:i32)
          n186 = Subtract(x=w470, y=w460) -> (x-y=w464:i32)
          n187 = Index Array(array=w467, index=w464) -> (element=w461:dbl)
          n188 = Index Array(array=w468, index=w464) -> (element=w469:dbl)
          n189 = Less?(x=w461, y=w466) -> (x < y?=w462:bool)
          n190 = Less Or Equal To 0?(x=w469) -> (x <= 0?=w463:bool)
          n191 = And(x=w462, y=w463) -> (x .and. y?=w465:bool)
        }
        n192 = Multiply(x=w338, y=w337) -> (x*y=w332:dbl[])
        n193 = Array Subset "P"(array=w332, length=w176) -> (w284:dbl[])  [unwired: 1 in]
        n194 = Increment(x=w331) -> (x+1=w178:i32)
        n195 = Array Subset "AFR"(array=w162, length=w176) -> (w165:dbl[])  [unwired: 1 in]
        n196 = Array Subset "EGT"(array=w163, length=w176) -> (w177:dbl[])  [unwired: 1 in]
        n197 = local read "Mv: M1 [Nm]"() -> (w216:dbl)
        n198 = local read "Mv: M0 [Nm]"() -> (w217:dbl)
        n199 = local read "Mv: n1 [1/min]"() -> (w215:u16)
        n200 = Array Subset "nWelle (Zündung)"(array=w238, index=w178) -> (w225:dbl[])  [unwired: 1 in]
        n201 = Array Subset "P"(array=w284, index=w178) -> (w173:dbl[])  [unwired: 1 in]
        n202 = Array Subset "n"(array=w242, index=w178) -> (w241:dbl[])  [unwired: 1 in]
        n203 = Array Subset "M"(array=w285, index=w178) -> (w271:dbl[])  [unwired: 1 in]
        n204 = Array Subset "AFR"(array=w165, index=w178) -> (w166:dbl[])  [unwired: 1 in]
        n205 = Array Subset "EGT"(array=w177, index=w178) -> (w161:dbl[])  [unwired: 1 in]
        n206 = Array Max & Min "nmax [1/min]"(array=w241) -> (max value=w313:dbl)  [unwired: 3 out]
        n207 = Array Max & Min "Pmax"(array=w173) -> (max value=w275:dbl, max index (indices)=w226:i32)  [unwired: 2 out]
        n208 = Array Max & Min "Mmax"(array=w271) -> (max value=w223:dbl, max index (indices)=w261:i32)  [unwired: 2 out]
        n209 = local read "air pressure [mbar]"() -> (w219:dbl)
        n210 = local read "air temp. [°C]"() -> (w220:dbl)
        n211 = local read "n min [1/min]"() -> (w269:dbl)
        n212 = local read "v min [km/h]"() -> (w268:dbl)
        n213 = Index Array "n(Mmax)"(array=w241, index=w261) -> (element=w222:dbl)
        n214 = Index Array "n(Pmax)"(array=w241, index=w226) -> (element=w230:dbl)
        n215 = Index Array "nWelle (Zündung) (Pmax)"(array=w225, index=w226) -> (element=w224:dbl)
        n216 = Divide(x=w313, y=w211) -> (x/y=w228:dbl)
        n217 = local read "Übersetzung ermitteln aus"() -> (w277:T2)
        n218 = Bundle By Name(cluster=w320, "Fahrzeugdaten"=w189, "Auto-Pfad"=w218, "Rolle [Inkr/U]"=w319, "Rollenumfang [m]"=w229, "Rollenträgheit [kgm²]"="inertia dyno [kgm²]", "Zündung [Imp/U]"=w316, "Getriebe [1:]"=w315, "Reifenumfang [m]"=w314, "element"=w211, "Gl. Mittelwert"="mov. Average", "Differenzenquotient"="diff.quotient", "dT [s]"=w286, "Strecke [m]"=w190, "Lufttemperatur [°C]"=w220, "Mv: n1 [1/min]"=w215, "Luftdruck [mbar]"=w219, "Übersetzung ermitteln aus"=w246, "[s]"=w312, "Mv: M0 [Nm]"=w217, "Mv: M1 [Nm]"=w216, "n vom Gas [1/min]"=w269, "Boolesch"=w317, "Serielle Schnittstelle"=refnum<visa-resource-name> refnum, "nKuWe/nRolle 2"=w270, "v vom Gas [km/h]"=w268) -> (w310:T3)
        n219 = Format Into String(format string="%.1f PS" ("Format-String"), w275) -> (resulting string=→"Pmax":string)  [unwired: 2 in, 1 out]
        n220 = case shown="Standard" w277 {
          tunnel: w229 -> [_ w391]
          tunnel: w241 -> [w381 w390]
          tunnel: [w381 w387] -> w180
          tunnel: [TRUE FALSE] -> w272
          tunnel: ["n [1/min]" "v [km/h]"] -> w181
          tunnel: w271 -> [w378 _]
          tunnel: [w378 w383] -> w179
          tunnel: [w374 w382] -> w251
          tunnel: w225 -> [_ w383]
          tunnel: [w375 w384] -> w250
          tunnel: w223 -> [w375 _]
          tunnel: [w374 w382] -> w249
          frame Default {
            w374 = "M [Nm]"
            n221 = property on="n min [1/min]" class="DigWert (strikt)"("DisabledEnum"=T5."Enabled" ("Deaktiviert")) -> ()  [unwired: 2 in, 2 out]
            n222 = property on="v min [km/h]" class="DigWert (strikt)"("DisabledEnum"=T5."Disabled and Grayed Out" ("Deaktiviert")) -> ()  [unwired: 2 in, 2 out]
          }
          frame "vario [km/h]" {
            w382 = "n [1/min]"
            n223 = Compound Arithmetic op=MULTIPLY(w390, w391, 0.06) -> (w387:dbl[])
            n224 = property on="v min [km/h]" class="DigWert (strikt)"("DisabledEnum"=T5."Enabled" ("Deaktiviert")) -> ()  [unwired: 2 in, 2 out]
            n225 = property on="n min [1/min]" class="DigWert (strikt)"("DisabledEnum"=T5."Disabled and Grayed Out" ("Deaktiviert")) -> ()  [unwired: 2 in, 2 out]
            n226 = Array Max & Min "nmax"(array=w383) -> (max value=w384:dbl)  [unwired: 3 out]
          }
        }
        "CursorX - Beschriftung" <- w181
        "CursorY2 - Beschriftung" <- w249
        n227 = Compound Arithmetic op=MULTIPLY "v(Pmax)"(w229, w230, w227) -> (w274:dbl)
        n228 = Compound Arithmetic op=MULTIPLY "vmax"(w229, w228, w227) -> (w221:dbl)
        n229 = Greater?(x=w190, y=2.0) -> (0:w199:bool)
        n230 = Format Into String(format string="   |   %.0f m\\n" ("Format-String"), w190) -> (resulting string=w197:string)  [unwired: 2 in, 1 out]
        n231 = Select(t=w197, s=w199, f="\r\n") -> (s? t:f=w193:string)
        n232 = Format Into String(format string="%.1f PS bei %d 1/min   |   %.1f Nm bei %d 1/min   |   vmax: %d km/h\\nDIN 70020 k =%.3f (%d \\B0C, %d mbar)" ("Format-String"), w275, w230, w223, w222, w221, w201, w220, w219) -> (resulting string=w231:string)  [unwired: 2 in, 1 out]
        n233 = Format Into String(format string="%.1f PS bei %d km/h, %d 1/min   |   vmax: %d km/h\\nDIN 70020 k =%.3f (%d \\B0C, %d mbar)" ("Format-String"), w275, w274, w224, w221, w201, w220, w219) -> (resulting string=w232:string)  [unwired: 2 in, 1 out]
        n234 = local read "Lambda"() -> (w168:bool)
        n235 = Select(t=0.06802721088435, s=w168, f=1.0) -> (s? t:f=w171:dbl)
        n236 = Multiply(x=w171, y=w166) -> (x*y=w167:dbl[])
        n237 = local read "Datum+Zeit"() -> (w205:string)
        n238 = local read "Dateiname"() -> (w196:string)
        n239 = Match Pattern(string=w205, regular expression=" $") -> (before substring=w194:string)  [unwired: 1 in, 3 out]
        n240 = Select(t=w231, s=w272, f=w232) -> (s? t:f=w207:string)
        n241 = Bundle(w180, w173) -> (w304:cluster{dbl[], dbl[]})  [unwired: 1 in]
        n242 = Bundle(w180, w179) -> (w303:cluster{dbl[], dbl[]})  [unwired: 1 in]
        n243 = Bundle(w180, w167) -> (w183:cluster{dbl[], dbl[]})  [unwired: 1 in]
        n244 = Bundle(w180, w161) -> (w184:cluster{dbl[], dbl[]})  [unwired: 1 in]
        n245 = property on="XY-Graph" class="XYGraph (strikt)"("ActYScl"=1, "YScale.NameLbl.Text"=w251, "XScale.NameLbl.Text"=w181) -> ()  [unwired: 2 in, 2 out]
        n246 = Concatenate Strings(w207, w193, w194, " | ", w196) -> (w206:string)
        n247 = Build Array(w304, w303) -> (w259:cluster{dbl[], dbl[]}[])
        n248 = Build Array(w183, w184) -> (w182:cluster{dbl[], dbl[]}[])
        n249 = flat-sequence {
          tunnel: [w398] -> w309
          tunnel: [w401] -> w307
          tunnel: [w400] -> w306
          tunnel: w259 -> [w397]
          tunnel: [w396] -> w258
          tunnel: w189 -> [w399]
          tunnel: w310 -> [w402]
          tunnel: w206 -> [w403]
          tunnel: [w395] -> w185
          tunnel: w182 -> [w394]
          tunnel: [w426] -> w187
          tunnel: [w427] -> w308
          tunnel: w307 -> [w427]
          tunnel: w306 -> [w426]
          tunnel: [w424] -> w257
          tunnel: w258 -> [w424]
          tunnel: w185 -> [w423]
          tunnel: [w423] -> w172
          frame #0 {
            n250 = local read "Überlagerung"() -> (w398:bool)
            n251 = case shown="False" w398 {
              tunnel: w403 -> [w408 w421]
              tunnel: [w408 w422] -> w401
              tunnel: w402 -> [w407 _]
              tunnel: w399 -> [w406 w419]
              tunnel: [w406 w418] -> w400
              tunnel: w397 -> [w405 w413]
              tunnel: [w405 w412] -> w396
              tunnel: w394 -> [w404 w410]
              tunnel: [w404 w409] -> w395
              frame False {
                n252 = local write "Datenspeicher"(w407) -> ()
              }
              frame True {
                w417 = "\t"
                w420 = "\n"
                n253 = local read "Fahrzeugdaten"() -> (w416:string)
                n254 = local read "AFR,EGT-Graph"() -> (w411:cluster{dbl[], dbl[]}[])
                n255 = local read "XY-Graph"() -> (w414:cluster{dbl[], dbl[]}[])
                n256 = local read "Ergebnis"() -> (w415:string)
                n257 = Concatenate Strings(w416, w417, w420, w419) -> (w418:string)
                n258 = Concatenate Strings(w415, w417, w420, w421) -> (w422:string)
                n259 = Insert Into Array(array=w414, new element=w413) -> (w412:cluster{dbl[], dbl[]}[])  [unwired: 1 in]
                n260 = Insert Into Array(array=w411, new element=w410) -> (w409:cluster{dbl[], dbl[]}[])  [unwired: 1 in]
              }
            }
          }
          frame #1 {
            n261 = Wait (ms)(milliseconds to wait=u32 0 ("Zu wartende ms")) -> ()  [unwired: 1 out]
          }
        }
        n262 = property on="AFR,EGT-Graph" class="XYGraph (strikt)"("XScale.NameLbl.Text"=w181) -> ()  [unwired: 2 in, 2 out]
        n263 = Search/Split String "Überschrift\nwegschneiden"(string=w187, search string/char (-)="§$") -> (substring before match=→"Fahrzeugdaten":string)  [unwired: 1 in, 2 out]
        n264 = Array Size(array=w257) -> (size(s)=w191:i32)
        n265 = Multiply(x=w250, y=1.8) -> (x*y=w281:dbl)
        n266 = flat-sequence {
          tunnel: w191 -> [w359]
          tunnel: w190 -> [w350]
          frame #0 {
            w353 = refnum<vi> refnum  # Numerisch
            n267 = control-ref of="Strecken"() -> (w356:refnum<vi>)
            n268 = property on="Eigenschaftsknoten" class="Cluster (strikt)"(reference=w356) -> (error out=w354:errorcluster, "Controls[]"=w349:refnum<vi>[])  [unwired: 1 in, 1 out]
            n269 = Divide(x=w359, y=2) -> (x/y=w358:dbl)
            n270 = Decrement(x=w358) -> (x-1=w357:dbl)
            n271 = Index Array(array=w349, index=w357) -> (element=w355:refnum<vi>)
            n272 = To More Specific Class(target class=w353, reference=w355, error in=w354) -> (specific class reference=w352:refnum<vi>, error out=w351:errorcluster)
            n273 = property class="Num"(reference=w352, error in=w351, "Value"=w350) -> ()  [unwired: 2 out]
          }
          frame #1 {
            w362 = 100.0
            n274 = local read "Strecken"() -> (w367:T1)
            n275 = Cluster To Array(cluster=w367) -> (array=w366:dbl[])
            n276 = Array Max & Min(array=w366) -> (max value=w365:dbl)  [unwired: 3 out]
            n277 = Quotient & Remainder(x=w365, y=w362) -> (floor(x/y)=w364:dbl)  [unwired: 1 out]
            n278 = Increment(x=w364) -> (x+1=w363:dbl)
            n279 = Multiply(x=w363, y=w362) -> (x*y=w361:dbl)
            n280 = property on="Strecke1" class="Schieber (strikt)"("Scale.Maximum"=w361) -> ()  [unwired: 2 in, 2 out]
            n281 = property on="Strecke2" class="Schieber (strikt)"("Scale.Maximum"=w361) -> ()  [unwired: 2 in, 2 out]
            n282 = property on="Strecke6" class="Schieber (strikt)"("Scale.Maximum"=w361) -> ()  [unwired: 2 in, 2 out]
            n283 = property on="Strecke3" class="Schieber (strikt)"("Scale.Maximum"=w361) -> ()  [unwired: 2 in, 2 out]
            n284 = property on="Strecke7" class="Schieber (strikt)"("Scale.Maximum"=w361) -> ()  [unwired: 2 in, 2 out]
            n285 = property on="Strecke4" class="Schieber (strikt)"("Scale.Maximum"=w361) -> ()  [unwired: 2 in, 2 out]
            n286 = property on="Strecke5" class="Schieber (strikt)"("Scale.Maximum"=w361) -> ()  [unwired: 2 in, 2 out]
          }
        }
        n287 = case shown="True" w309 {
          tunnel: w191 -> [_ w437]
          tunnel: w308 -> [_ w434]
          tunnel: w187 -> [_ w433]
          frame False {
            w428 = 1
            w430 = 0
            w429 = TRUE ("Plot.Sichtbar")
            w431 = u32 16711680
            n288 = property on="Fahrzeugdaten" class="Str"("Text.Font:Color"=w431) -> ()  [unwired: 2 in, 2 out]
            n289 = property on="Ergebnis" class="Str"("Text.Font:Color"=w431) -> ()  [unwired: 2 in, 2 out]
            n290 = property on="XY-Graph" class="XYGraph (strikt)"("Active Plot"=w430, "Plot.Visible?"=w429, "Active Plot"=w428, "Plot.Visible?"=w429) -> ()  [unwired: 2 in, 2 out]
            n291 = property on="AFR,EGT-Graph" class="XYGraph (strikt)"("Active Plot"=w430, "Plot.Visible?"=w429, "Active Plot"=w428, "Plot.Visible?"=w429) -> ()  [unwired: 2 in, 2 out]
          }
          frame True {
            w432 = 0
            n292 = for {
              N: w437 -> [_]
              shift-right: [w455] -> w435
              shift-left: u32[] [] -> [w454]
              i -> [w449]
              w453 = 2 ("y")
              n293 = Quotient & Remainder(x=w449, y=w453) -> (x-y*floor(x/y)=w446:i32)  [unwired: 1 out]
              n294 = Equal To 0?(x=w446) -> (x = 0?=w451:bool)
              n295 = Not Equal To 0?(x=w446) -> (x != 0?=w452:bool)
              n296 = Or(x=w451, y=w452) -> (x .or. y?=w448:bool)
              n297 = Select(t=w446, s=w451, f=w453) -> (s? t:f=w447:i32)
              n298 = property on="XY-Graph" class="XYGraph (strikt)"("Active Plot"=w449, "Plot.Visible?"=w448, "Plot.YScaleIdx"=w446, "Plot.Line Style"=w447) -> ("Plot.Plot Color"=w450:u32)  [unwired: 2 in, 2 out]
              n299 = property on="AFR,EGT-Graph" class="XYGraph (strikt)"("Active Plot"=w449, "Plot.Visible?"=w448, "Plot.YScaleIdx"=w446, "Plot.Line Style"=w447) -> ()  [unwired: 2 in, 2 out]
              n300 = case shown="True" w451 {
                tunnel: w450 -> [_ w459]
                tunnel: [w456 w458] -> w455
                tunnel: w454 -> [w456 w457]
                frame False {
                }
                frame True {
                  n301 = Insert Into Array(array=w457, new element=w459) -> (w458:u32[])  [unwired: 1 in]
                }
              }
            }
            n302 = for {
              shift-right: [w445] -> _
              shift-left: w432 -> [w442]
              tunnel: w435 -> [w443] mode=indexing
              tunnel: w434 -> [w444]
              tunnel: w433 -> [w441]
              shift-right: [w440] -> _
              shift-left: w432 -> [w439]
              w438 = "\t"
              n303 = Match Pattern(string=w441, regular expression=w438, offset (0)=w439) -> (offset past match=w440:i32)  [unwired: 3 out]
              n304 = Match Pattern(string=w444, regular expression=w438, offset (0)=w442) -> (offset past match=w445:i32)  [unwired: 3 out]
              n305 = property on="Fahrzeugdaten" class="Str"("Text.Selection Start"=w439, "Text.Selection End"=w440, "Text.FontColor"=w443) -> ()  [unwired: 2 in, 2 out]
              n306 = property on="Ergebnis" class="Str"("Text.Selection Start"=w442, "Text.Selection End"=w445, "Text.FontColor"=w443) -> ()  [unwired: 2 in, 2 out]
            }
          }
        }
        n307 = Round To Nearest(number=w281) -> (nearest integer value=w263:dbl)
        n308 = Max & Min(x=w191, y=2) -> (max(x,y)=w260:i32)  [unwired: 1 out]
        n309 = Greater Or Equal?(x=w191, y=14) -> (x >= y?=w301:bool)
        n310 = Multiply(x=w275, y=1.2) -> (x*y=w279:dbl)
        n311 = Round To Nearest(number=w279) -> (nearest integer value=w280:dbl)
        n312 = case shown="True" w301 {
          frame False {
          }
          frame True {
            n313 = property on="Überlagern" class="Bool. (strikt)"("DisabledEnum"=2) -> ()  [unwired: 2 in, 2 out]
          }
        }
        n314 = property on="XY-Graph" class="XYGraph (strikt)"("LegNumRows"=w260, "ActYScl"=1, "YScale.Maximum"=w263, "YScale.Minimum"=0) -> (error out=w254:errorcluster, "XScale.Minimum"=w175:dbl, "XScale.Maximum"=w174:dbl)  [unwired: 2 in, 1 out]
        n315 = property on="XY-Graph" class="XYGraph (strikt)"("ActYScl"=w262, "YScale.Maximum"=w280, "YScale.Minimum"=w262) -> ()  [unwired: 2 in, 2 out]
        n316 = Add(x=w175, y=w174) -> (x+y=w256:dbl)
        n317 = property on="AFR,EGT-Graph" class="XYGraph (strikt)"("XScale.Minimum"=w175, "XScale.Maximum"=w174) -> ()  [unwired: 2 in, 2 out]
        n318 = Divide(x=w256, y=2.0) -> (x/y=w253:dbl)
        n319 = property on="XY-Graph" class="XYGraph (strikt)"(error in=w254, "Active Cursor"=0, "Cursor.Cursor X"=w253) -> ("Width"=w160:u32)  [unwired: 1 in, 2 out]
        n320 = property on="AFR,EGT-Graph" class="XYGraph (strikt)"("Width"=w160) -> ()  [unwired: 2 in, 2 out]
        "Ergebnis" <- w308
        "XY-Graph" <- w257
        "AFR,EGT-Graph" <- w172
      }
      event "Speichern": Value Change {
        n321 = event-data() -> ("OldVal"=w516:bool)  [unwired: 1 in, 5 out]
        n322 = local write "Speichern"(w516) -> ()
        n323 = control-ref of="Datenspeicher"() -> (w515:refnum<vi>)
        n324 = call "SaveCluster (SubVI).vi"("Datenspeicher 2"=w515) -> ()  [unwired: 1 in, 1 out]
      }
      event "Stopp": Value Change {
        n325 = event-data() -> ("OldVal"=w517:bool, "NewVal"=w518:bool)  [unwired: 1 in, 4 out]
        n326 = local write "Stopp"(w517) -> ()
      }
      event "Legende einblenden": Value Change {
        n327 = event-data() -> ()  [unwired: 1 in, 6 out]
        n328 = local read "XY-Graph"() -> (w522:cluster{dbl[], dbl[]}[])
        n329 = Array Size(array=w522) -> (size(s)=w521:i32)
        n330 = Max & Min(x=w521, y=2) -> (max(x,y)=w519:i32)  [unwired: 1 out]
        n331 = property on="XY-Graph" class="XYGraph (strikt)"("Legend Visible"="Legende einblenden", "LegNumRows"=w519) -> ()  [unwired: 2 in, 2 out]
      }
      event "XY-Graph": Mouse Move {
        w541 = 0
        n332 = event-data() -> ()  [unwired: 1 in, 5 out]
        n333 = property on="XY-Graph" class="XYGraph (strikt)"("Active Cursor"=w541) -> (error out=w542:errorcluster, "Cursor.Cursor Plot"=w529:i32, "Cursor.Cursor X"=→"n [1/min]":dbl, "Cursor.Cursor Index"=w526:i32)  [unwired: 2 in, 1 out]
        n334 = Quotient & Remainder(x=w529, y=2) -> (x-y*floor(x/y)=w531:i32)  [unwired: 1 out]
        n335 = property on="XY-Graph" class="XYGraph (strikt)"(error in=w542, "Active Plot"=w529) -> (error out=w540:errorcluster, "Plot.Plot Color"=w525:u32)  [unwired: 1 in, 1 out]
        n336 = Equal To 0?(x=w531) -> (x = 0?=w530:bool)
        n337 = local read "AFR, EGT"() -> (w524:bool)
        n338 = case shown="True" w524 {
          tunnel: w530 -> [_ w556]
          tunnel: w529 -> [_ w555]
          tunnel: [w543 w548] -> w528
          tunnel: [w543 w544] -> w527
          tunnel: w526 -> [_ w547]
          frame False {
            w543 = 0.0
          }
          frame True {
            n339 = Decrement(x=w555) -> (x-1=w554:i32)
            n340 = Select(t=w555, s=w556, f=w554) -> (s? t:f=w553:i32)
            n341 = property on="AFR,EGT-Graph" class="XYGraph (strikt)"() -> ("Value"=w549:cluster{dbl[], dbl[]}[])  [unwired: 2 in, 2 out]
            n342 = Increment(x=w553) -> (x+1=w550:i32)
            n343 = Index Array(array=w549, index=w553) -> (element=w558:cluster{dbl[], dbl[]})
            n344 = Index Array(array=w549, index=w550) -> (element=w551:cluster{dbl[], dbl[]})
            n345 = Unbundle(w558) -> (w557:dbl[])  [unwired: 1 out]
            n346 = Unbundle(w551) -> (w552:dbl[])  [unwired: 1 out]
            n347 = Index Array(array=w557, index=w547) -> (element=w545:dbl)
            n348 = Index Array(array=w552, index=w547) -> (element=w548:dbl)
            n349 = local read "Lambda"() -> (w546:bool)
            n350 = case shown="False" w546 {
              tunnel: w545 -> [w560 w567]
              tunnel: [w559 w566] -> w544
              frame False {
                n351 = Greater?(x=w560, y=5.0) -> (0:w563:bool)
                n352 = Select(t=1.0, s=w563, f=14.7) -> (s? t:f=w561:dbl)
                n353 = Multiply(x=w560, y=w561) -> (x*y=w559:dbl)
              }
              frame True {
                n354 = Less?(x=w567, y=5.0) -> (x < y?=w570:bool)
                n355 = Select(t=1.0, s=w570, f=0.06802721088435375) -> (s? t:f=w568:dbl)
                n356 = Multiply(x=w567, y=w568) -> (x*y=w566:dbl)
              }
            }
          }
        }
        "AFR" <- w527
        "EGT [°C]" <- w528
        n357 = property on="n [1/min]" class="DigWert (strikt)"("NumText.TextColor"=w525) -> ()  [unwired: 2 in, 2 out]
        n358 = property on="P [PS]" class="DigWert (strikt)"("NumText.TextColor"=w525) -> ()  [unwired: 2 in, 2 out]
        n359 = property on="M [Nm]" class="DigWert (strikt)"("NumText.TextColor"=w525) -> ()  [unwired: 2 in, 2 out]
        n360 = property on="AFR" class="DigWert (strikt)"("NumText.TextColor"=w525) -> ()  [unwired: 2 in, 2 out]
        n361 = property on="EGT [°C]" class="DigWert (strikt)"("NumText.TextColor"=w525) -> ()  [unwired: 2 in, 2 out]
        n362 = property on="XY-Graph" class="XYGraph (strikt)"(error in=w540, "Active Cursor"=w541, "Cursor.Cursor Color"=w525) -> ()  [unwired: 1 in, 2 out]
        n363 = local read "Übersetzung ermitteln aus"() -> (w535:T2)
        n364 = property on="XY-Graph" class="XYGraph (strikt)"("Active Cursor"=0) -> ("Cursor.Cursor Y"=w533:dbl, "Cursor.Cursor X"=w532:dbl)  [unwired: 2 in, 2 out]
        n365 = case shown="True" w530 {
          tunnel: [w579 w596] -> w537
          tunnel: [w578 w595] -> w536
          tunnel: w535 -> [w577 w599]
          tunnel: w533 -> [w576 w598]
          tunnel: w532 -> [w575 w597]
          tunnel: w526 -> [w573 w594]
          tunnel: w529 -> [w574 w593]
          frame False {
            n366 = case shown="\"vario [km/h]\"" w577 {
              tunnel: [w582 w585] -> w579
              tunnel: [w581 w592] -> w578
              tunnel: w576 -> [w581 w592]
              tunnel: w575 -> [w580 _]
              tunnel: w574 -> [_ w587]
              tunnel: w573 -> [_ w586]
              frame Default {
                n367 = Multiply(x=w580, y=0.00014237924281946062) -> (x*y=w583:dbl)
                n368 = Multiply(x=w581, y=w583) -> (x*y=w582:dbl)
              }
              frame "vario [km/h]" {
                n369 = Decrement(x=w587) -> (x-1=w590:i32)
                n370 = local read "XY-Graph"() -> (w591:cluster{dbl[], dbl[]}[])
                n371 = Index Array(array=w591, index=w590) -> (element=w589:cluster{dbl[], dbl[]})
                n372 = Unbundle(w589) -> (w588:dbl[])  [unwired: 1 out]
                n373 = Index Array(array=w588, index=w586) -> (element=w585:dbl)
              }
            }
          }
          frame True {
            n374 = case shown="\"vario [km/h]\"" w599 {
              tunnel: w598 -> [w601 w607]
              tunnel: w597 -> [w602 _]
              tunnel: [w601 w607] -> w596
              tunnel: [w600 w606] -> w595
              tunnel: w594 -> [_ w608]
              tunnel: w593 -> [_ w612]
              frame Default {
                w603 = 7023.495702024609  # 60/(2Pi) * W/PS
                n375 = Divide(x=w603, y=w602) -> (x/y=w604:dbl)
                n376 = Multiply(x=w601, y=w604) -> (x*y=w600:dbl)
              }
              frame "vario [km/h]" {
                n377 = Increment(x=w612) -> (x+1=w610:i32)
                n378 = local read "XY-Graph"() -> (w611:cluster{dbl[], dbl[]}[])
                n379 = Index Array(array=w611, index=w610) -> (element=w609:cluster{dbl[], dbl[]})
                n380 = Unbundle(w609) -> (w605:dbl[])  [unwired: 1 out]
                n381 = Index Array(array=w605, index=w608) -> (element=w606:dbl)
              }
            }
          }
        }
        "M [Nm]" <- w536
        "P [PS]" <- w537
      }
      event "AFR, EGT": Value Change {
        w621 = 2  # Deaktivieren
        w620 = 0  # Aktivieren
        n382 = event-data() -> ("NewVal"=w616:bool)  [unwired: 1 in, 5 out]
        n383 = local read "Höhe Leistungs-Graph (646)"() -> (w625:u32)
        n384 = local read "Y-Koord. Leistungsgraph-Reset-Button unten (782)"() -> (w617:i32)
        n385 = local read "Y-Koord. Leistungsgraph-Reset-Button oben (567)"() -> (w618:i32)
        n386 = control-ref of="AFR,EGT-Graph"() -> (w622:refnum<vi>)
        n387 = control-ref of="XY-Graph"() -> (w624:refnum<vi>)
        n388 = call "ReCalc - Enable_AFR_EGT_Graph (SubVI).vi"("Leistungsgraph"=w624, "AFR EGT"=w616, "Höhe Leistungs-Graph"=w625, "AFR EGT Gaph"=w622, "Skalierungsfaktor Leistungsgraph"=0.6666666666666666) -> ()  [unwired: 11 in]
        n389 = Select(t=w618, s=w616, f=w617) -> (s? t:f=w613:i32)
        n390 = property on="Autoskalierung Leistung" class="Bool. (strikt)"("Top"=w613) -> ("Height"=w614:u32)  [unwired: 2 in, 2 out]
        n391 = property on="Legende einblenden" class="Bool. (strikt)"("Top"=w613) -> ()  [unwired: 2 in, 2 out]
        n392 = Add(x=w614, y=w613) -> (x+y=w615:u32)
        n393 = property on="Resetskalierung Leistung" class="Bool. (strikt)"("Top"=w615) -> ()  [unwired: 2 in, 2 out]
        n394 = Select(t=w620, s=w616, f=w621) -> (s? t:f=w619:i32)
        n395 = property on="CursorAFR - Beschriftung" class="Str"("DisabledEnum"=w619) -> ()  [unwired: 2 in, 2 out]
        n396 = property on="EGT [°C]" class="DigWert (strikt)"("DisabledEnum"=w619) -> ()  [unwired: 2 in, 2 out]
        n397 = property on="Autoskalierung AFR" class="Bool. (strikt)"("Visible"=w616) -> ()  [unwired: 2 in, 2 out]
        n398 = property on="AFR" class="DigWert (strikt)"("DisabledEnum"=w619) -> ()  [unwired: 2 in, 2 out]
        n399 = property on="Resetskalierung AFR" class="Bool. (strikt)"("Visible"=w616) -> ()  [unwired: 2 in, 2 out]
      }
      event "Lambda": Value Change {
        w636 = 0
        n400 = event-data() -> ("NewVal"=w628:bool)  [unwired: 1 in, 5 out]
        n401 = local read "AFR"() -> (w627:dbl)
        n402 = local read "AFR,EGT-Graph"() -> (w633:cluster{dbl[], dbl[]}[])
        n403 = case shown="True" w628 {
          tunnel: ["AFR" "l"] -> w631
          tunnel: ["Anwendung" "Symbol"] -> w632
          tunnel: [20.0 1.6] -> w647
          tunnel: [10.0 0.4] -> w645
          tunnel: [w683 w688] -> w646
          tunnel: [w683 w688] -> w629
          frame False {
            w683 = 1
          }
          frame True {
            w688 = 2
          }
        }
        n404 = case shown="False" w628 {
          tunnel: w627 -> [w649 w656]
          tunnel: [w648 w655] -> w626
          frame False {
            n405 = Greater?(x=w649, y=5.0) -> (0:w652:bool)
            n406 = Select(t=1.0, s=w652, f=14.7) -> (s? t:f=w650:dbl)
            n407 = Multiply(x=w649, y=w650) -> (x*y=w648:dbl)
          }
          frame True {
            n408 = Less?(x=w656, y=5.0) -> (x < y?=w659:bool)
            n409 = Select(t=1.0, s=w659, f=0.06802721088435375) -> (s? t:f=w657:dbl)
            n410 = Multiply(x=w656, y=w657) -> (x*y=w655:dbl)
          }
        }
        n411 = Array Size(array=w633) -> (size(s)=w635:i32)
        n412 = for {
          N: w635 -> [_]
          tunnel: w628 -> [w664]
          shift-right: [w662] -> w634
          shift-left: w633 -> [w663]
          i -> [w665]
          n413 = Quotient & Remainder(x=w665, y=2) -> (x-y*floor(x/y)=w667:i32)  [unwired: 1 out]
          n414 = Equal To 0? "AFR-Plot?"(x=w667) -> (x = 0?=w666:bool)
          n415 = case shown="True" w666 {
            tunnel: w665 -> [_ w673]
            tunnel: w664 -> [_ w675]
            tunnel: w663 -> [w669 w670]
            tunnel: [w669 w671] -> w662
            frame False {
            }
            frame True {
              n416 = Index Array(array=w670, index=w673) -> (element=w672:cluster{dbl[], dbl[]})
              n417 = Unbundle(w672) -> (w679:dbl[], w676:dbl[])
              n418 = Multiply(x=0.06802721088435375, y=w676) -> (x*y=w682:dbl[])
              n419 = Multiply(x=14.7, y=w676) -> (x*y=w681:dbl[])
              n420 = Select(t=w682, s=w675, f=w681) -> (s? t:f=w680:dbl[])
              n421 = Bundle(w679, w680) -> (w674:cluster{dbl[], dbl[]})  [unwired: 1 in]
              n422 = Replace Array Subset(array=w670, new element=w674, index=w673) -> (w671:cluster{dbl[], dbl[]}[])
            }
          }
        }
        n423 = property on="AFR,EGT-Graph" class="XYGraph (strikt)"("ActYScl"=w636, "YScale.NameLbl.Text"=w631, "YScale.NameLbl.FontName"=w632, "YScale.Maximum"=w647, "YScale.Minimum"=w645, "YScale.Precision"=w646) -> ("Height"=w639:u32, "YScale.NameLbl.Width"=w638:u32, "Top"=w637:i32)  [unwired: 2 in, 2 out]
        n424 = property on="CursorAFR - Beschriftung" class="Str"("Text.Text"=w631, "Text.FontName"=w632) -> ()  [unwired: 2 in, 2 out]
        n425 = property on="AFR" class="DigWert (strikt)"("Format"=0, "Precision"=w629, "Value"=w626) -> ()  [unwired: 2 in, 2 out]
        n426 = Subtract(x=w639, y=w638) -> (x-y=w640:u32)
        n427 = Divide(x=w640, y=2) -> (x/y=w642:dbl)
        n428 = Add(x=w642, y=w637) -> (x+y=w643:dbl)
        n429 = property on="AFR,EGT-Graph" class="XYGraph (strikt)"("ActYScl"=w636, "YScale.NameLbl.Top"=w643, "Active Plot"=0) -> ()  [unwired: 2 in, 2 out]
        n430 = property on="AFR,EGT-Graph" class="XYGraph (strikt)"("Value"=w634) -> ()  [unwired: 2 in, 2 out]
      }
      event "XY-Graph": Mouse Up {
        n431 = event-data() -> ()  [unwired: 1 in, 8 out]
        n432 = local read "XY-Graph"() -> (w694:cluster{dbl[], dbl[]}[])
        n433 = Array Size(array=w694) -> (size(s)=w693:i32)
        n434 = for {
          N: w693 -> [_]
          i -> [w700]
          n435 = Quotient & Remainder(x=w700, y=2) -> (x-y*floor(x/y)=w702:i32)  [unwired: 1 out]
          n436 = Equal To 0?(x=w702) -> (x = 0?=w701:bool)
          n437 = case shown="True" w701 {
            tunnel: w700 -> [w704 w706]
            tunnel: [w704 w706] -> w696
            tunnel: [w705 w707] -> w695
            frame False {
              n438 = Decrement(x=w704) -> (x-1=w705:i32)
            }
            frame True {
              n439 = Increment(x=w706) -> (x+1=w707:i32)
            }
          }
          n440 = property on="XY-Graph" class="XYGraph (strikt)"("Active Plot"=w696, "Active Plot"=w695) -> ("Plot.Visible?"=w699:bool, "Plot.Visible?"=w698:bool)  [unwired: 2 in, 2 out]
          n441 = Or(x=w699, y=w698) -> (x .or. y?=w697:bool)
          n442 = property on="AFR,EGT-Graph" class="XYGraph (strikt)"("Active Plot"=w696, "Plot.Visible?"=w697, "Active Plot"=w695, "Plot.Visible?"=w697) -> ()  [unwired: 2 in, 2 out]
        }
      }
      event "Autoskalierung Leistung": Value Change {
        w710 = 1  # Einmalige Autoskalierung
        n443 = event-data() -> ()  [unwired: 1 in, 6 out]
        n444 = property on="XY-Graph" class="XYGraph (strikt)"("ActYScl"=0, "YScale.ScaleFit"=w710, "ActYScl"=1, "YScale.ScaleFit"=w710, "XScale.ScaleFit"=w710) -> ("XScale.Maximum"=w709:dbl, "XScale.Minimum"=w708:dbl)  [unwired: 2 in, 2 out]
        n445 = property on="AFR,EGT-Graph" class="XYGraph (strikt)"("XScale.Maximum"=w709, "XScale.Minimum"=w708) -> ()  [unwired: 2 in, 2 out]
      }
      event "Autoskalierung AFR": Value Change {
        w715 = 1  # Einmalige Autoskalierung
        n446 = event-data() -> ()  [unwired: 1 in, 6 out]
        n447 = property on="AFR,EGT-Graph" class="XYGraph (strikt)"("ActYScl"=0, "YScale.ScaleFit"=w715, "ActYScl"=1, "YScale.ScaleFit"=w715, "XScale.ScaleFit"=w715) -> ("XScale.Maximum"=w714:dbl, "XScale.Minimum"=w713:dbl)  [unwired: 2 in, 2 out]
        n448 = property on="XY-Graph" class="XYGraph (strikt)"("XScale.Maximum"=w714, "XScale.Minimum"=w713) -> ()  [unwired: 2 in, 2 out]
      }
      event "Resetskalierung AFR": Value Change {
        n449 = event-data() -> ()  [unwired: 1 in, 6 out]
        n450 = local read "Lambda"() -> (w725:bool)
        n451 = case shown="True" w725 {
          tunnel: [20.0 1.6] -> w724
          tunnel: [10.0 0.4] -> w723
          frame False {
          }
          frame True {
          }
        }
        n452 = property on="AFR,EGT-Graph" class="XYGraph (strikt)"("ActYScl"=0, "YScale.Maximum"=w724, "YScale.Minimum"=w723, "ActYScl"=1, "YScale.Maximum"=800.0, "YScale.Minimum"=0.0, "XScale.ScaleFit"=1) -> ("XScale.Maximum"=w719:dbl, "XScale.Minimum"=w718:dbl)  [unwired: 2 in, 2 out]
        n453 = property on="XY-Graph" class="XYGraph (strikt)"("XScale.Maximum"=w719, "XScale.Minimum"=w718) -> ()  [unwired: 2 in, 2 out]
      }
      event "Resetskalierung Leistung": Value Change {
        w736 = 0
        n454 = event-data() -> ()  [unwired: 1 in, 6 out]
        n455 = local read "Übersetzung ermitteln aus"() -> (w739:T2)
        n456 = case shown="\"vario [km/h]\"" w739 {
          tunnel: [50.0 14000.0] -> w735
          frame Default {
          }
          frame "vario [km/h]" {
          }
        }
        n457 = property on="XY-Graph" class="XYGraph (strikt)"("ActYScl"=w736, "YScale.Maximum"=30.0, "YScale.Minimum"=w736, "ActYScl"=1, "YScale.Maximum"=w735, "YScale.Minimum"=w736, "XScale.ScaleFit"=1) -> ("XScale.Maximum"=w733:dbl, "XScale.Minimum"=w732:dbl)  [unwired: 2 in, 2 out]
        n458 = property on="AFR,EGT-Graph" class="XYGraph (strikt)"("XScale.Maximum"=w733, "XScale.Minimum"=w732) -> ()  [unwired: 2 in, 2 out]
      }
    }
  }
  n459 = property on="Fensterbereich" class="Bereich"("Origin"=T4 {"Horizontal"=8, "Vertical"=6}) -> ()  [unwired: 2 in, 2 out]
  n460 = case shown="True" "Berechnen" {
    selector: "Berechnen" -> [_ w745]
    frame False {
    }
    frame True {
      n461 = property on="Berechnen" class="Bool. (strikt)"("Value"=w745, "DisabledEnum"=T5."Enabled" ("Deaktiviert")) -> (error out=w742:errorcluster)  [unwired: 2 in, 1 out]
      n462 = property on="Öffnen" class="Bool. (strikt)"(error in=w742, "Val(Sgnl)"=TRUE ("Wert (signalisierend)")) -> ()  [unwired: 1 in, 2 out]
    }
  }
  n463 = property on="Berechnen" class="Bool. (strikt)"("DisabledEnum"=w9) -> ()  [unwired: 2 in, 2 out]
  n464 = property on="Überlagern" class="Bool. (strikt)"("DisabledEnum"=w9) -> ()  [unwired: 2 in, 2 out]
  n465 = property on="Speichern" class="Bool. (strikt)"("DisabledEnum"=w9) -> ()  [unwired: 2 in, 2 out]
  n466 = property on="Drucken" class="Bool. (strikt)"("DisabledEnum"=w9) -> ()  [unwired: 2 in, 2 out]
  n467 = property on="CursorAFR - Beschriftung" class="Str"("DisabledEnum"=w9) -> ()  [unwired: 2 in, 2 out]
  n468 = property on="EGT [°C]" class="DigWert (strikt)"("DisabledEnum"=w9) -> ()  [unwired: 2 in, 2 out]
  n469 = property on="AFR" class="DigWert (strikt)"("DisabledEnum"=w9) -> ()  [unwired: 2 in, 2 out]
  n470 = property on="Lambda" class="Bool. (strikt)"("Value"=FALSE) -> ()  [unwired: 2 in, 2 out]
  n471 = property on="AFR, EGT" class="Bool. (strikt)"("Value"=FALSE) -> ()  [unwired: 2 in, 2 out]
  n472 = property on="Überlagerung" class="Bool. (strikt)"("Value"=FALSE) -> ()  [unwired: 2 in, 2 out]
  n473 = property on="mov. Average" class="DigWert (strikt)"("DisabledEnum"=w29) -> ()  [unwired: 2 in, 2 out]
  n474 = property on="diff.quotient" class="DigWert (strikt)"("DisabledEnum"=w29) -> ()  [unwired: 2 in, 2 out]
  n475 = property on="Ergebnis" class="Str"("Value"=w26) -> ()  [unwired: 2 in, 2 out]
  n476 = property on="Pmax" class="Str"("Value"=w26) -> ()  [unwired: 2 in, 2 out]
  n477 = property on="Fahrzeugdaten" class="Str"("Value"=w26) -> ()  [unwired: 2 in, 2 out]
  n478 = property on="Dateiname" class="Str"("Value"=w26) -> ()  [unwired: 2 in, 2 out]
  n479 = property on="title diagram" class="Str"("Value"=w26) -> ()  [unwired: 2 in, 2 out]
  n480 = property on="Mv: M0 [Nm]" class="DigWert (strikt)"("DisabledEnum"=w29) -> ()  [unwired: 2 in, 2 out]
  n481 = property on="Mv: n1 [1/min]" class="DigWert (strikt)"("DisabledEnum"=w29) -> ()  [unwired: 2 in, 2 out]
  n482 = property on="Mv: M1 [Nm]" class="DigWert (strikt)"("DisabledEnum"=w29) -> ()  [unwired: 2 in, 2 out]
  n483 = local read "Höhe Leistungs-Graph (646)"() -> (w13:u32)
  n484 = property on="M [Nm]" class="DigWert (strikt)"("Value"=w10) -> ()  [unwired: 2 in, 2 out]
  n485 = property on="n [1/min]" class="DigWert (strikt)"("Value"=w10) -> ()  [unwired: 2 in, 2 out]
  n486 = Bundle(w33, w33) -> (w32:cluster{dbl[], dbl[]})  [unwired: 1 in]
  n487 = property on="P [PS]" class="DigWert (strikt)"("Value"=w10) -> ()  [unwired: 2 in, 2 out]
  n488 = property on="AFR" class="DigWert (strikt)"("Value"=w10) -> ()  [unwired: 2 in, 2 out]
  n489 = property on="EGT [°C]" class="DigWert (strikt)"("Value"=w10) -> ()  [unwired: 2 in, 2 out]
  n490 = Bundle(w27, w27, w27, w27, w27, w27, w27) -> (→"Strecken":cluster{dbl, dbl, dbl, dbl, dbl, dbl, dbl})  [unwired: 1 in]
  n491 = Build Array(w32, w32) -> (w25:cluster{dbl[], dbl[]}[])
  n492 = property on="XY-Graph" class="XYGraph (strikt)"("Value"=w25, "Active Cursor"=w31, "Cursor.Cursor Color"=w31, "Legend Visible"=TRUE, "LegNumRows"=2, "Height"=w13) -> ("Width"=w2:u32)  [unwired: 2 in, 2 out]
  n493 = property on="AFR,EGT-Graph" class="XYGraph (strikt)"("Value"=w25, "ActYScl"=0, "YScale.NameLbl.Text"=w12, "YScale.NameLbl.FontName"=w11, "YScale.Maximum"=20.0, "YScale.Minimum"=10.0, "YScale.ScaleFit"=w14, "ActYScl"=1, "YScale.Maximum"=800.0, "YScale.Minimum"=0.0, "YScale.ScaleFit"=w14, "XScale.ScaleFit"=w14, "Width"=w2) -> ()  [unwired: 2 in, 2 out]
  n494 = local read "Y-Koord. Leistungsgraph-Reset-Button unten (782)"() -> (w1:i32)
  n495 = property on="P [PS]" class="DigWert (strikt)"("NumText.TextColor"=w8) -> ()  [unwired: 2 in, 2 out]
  n496 = property on="AFR" class="DigWert (strikt)"("NumText.TextColor"=w8) -> ()  [unwired: 2 in, 2 out]
  n497 = property on="EGT [°C]" class="DigWert (strikt)"("NumText.TextColor"=w8) -> ()  [unwired: 2 in, 2 out]
  n498 = property on="M [Nm]" class="DigWert (strikt)"("NumText.TextColor"=w8) -> ()  [unwired: 2 in, 2 out]
  n499 = property on="n [1/min]" class="DigWert (strikt)"("NumText.TextColor"=w8) -> ()  [unwired: 2 in, 2 out]
  n500 = property on="CursorAFR - Beschriftung" class="Str"("Text.FontName"=w11) -> ()  [unwired: 2 in, 2 out]
  n501 = property on="AFR" class="DigWert (strikt)"("Format"=0, "Precision"=1) -> ()  [unwired: 2 in, 2 out]
  n502 = property on="Autoskalierung AFR" class="Bool. (strikt)"("Visible"=w5) -> ()  [unwired: 2 in, 2 out]
  n503 = property on="Resetskalierung AFR" class="Bool. (strikt)"("Visible"=w5) -> ()  [unwired: 2 in, 2 out]
  n504 = property on="Autoskalierung Leistung" class="Bool. (strikt)"("Top"=w1) -> ("Height"=w3:u32)  [unwired: 2 in, 2 out]
  n505 = property on="Legende einblenden" class="Bool. (strikt)"("Top"=w1) -> ()  [unwired: 2 in, 2 out]
  n506 = Add(x=w3, y=w1) -> (x+y=w4:u32)
  n507 = property on="Resetskalierung Leistung" class="Bool. (strikt)"("Top"=w4) -> ()  [unwired: 2 in, 2 out]
  "CursorAFR - Beschriftung" <- w12
